vi "dI-dV(V)_two devices_MFLI_MF-MD_K3636B_PK_V4.0_Ja.vi"() -> ()   [LabVIEW 2016]
uses:
  <instrlib>/Keithley 2600 Series/Public/Configure/Source/Configure Source (Limit).vi
  <instrlib>/Keithley 2600 Series/Public/Configure/Source/Configure Source (Range).vi
  <instrlib>/Zurich Instruments LabOne/Public/Configure/ziSetValueDouble.vi
  <instrlib>/Zurich Instruments LabOne/Public/Configure/ziGetValueDemodSampleEx.vi
  <instrlib>/Zurich Instruments LabOne/Zurich Instruments LabOne.lvlib
  <instrlib>/Keithley 2600 Series/Keithley 2600 Series.lvlib
panel:
  in  "MFLI autorange":bool
  in  "MFLI autophase":bool=TRUE
  out "data 2":dbl[](array[numeric])=[5031.359, -0.0019808823515, 7.18983667949342e-11, 8.223089583294991e-06, 8.743473613736861e-06, -0.30000000000000016, -1.500000000000001e-08]
  in  "Tab Control":enum32{"Device 1", "Device 2"}(tab)
  out "dI/dV vs DC Bias (Device 1)":cluster{dbl, "Field Reading":dbl}[](graph)=[{-0.0016781686070000002, "Field Reading"=2.2748202419571386e-06}, {-0.0016578232874999998, "Field Reading"=2.3367028842127987e-06}, {-0.0016344170475, "Field Reading"=2.3324300158885588e-06}, {-0.0016187565549999998, "Field Reading"=2.368210290712901e-06}, {-0.0015966937695, "Field Reading"=2.4050914536005733e-06}, {-0.0015758724415, "Field Reading"=2.462219692201584e-06}, {-0.001552636935, "Field Reading"=2.492132794862598e-06}, {-0.0015335452565, "Field Reading"=2.4689307008136067e-06}, {-0.0015116246024999998, "Field Reading"=2.4182849093288775e-06}, {-0.0014938772125, "Field Reading"=2.3712011536684357e-06}, {-0.001474904835, "Field Reading"=2.336630295077755e-06}, {-0.0014527027135000001, "Field Reading"=2.3489588007080005e-06}, {-0.001433562216, "Field Reading"=2.4000938479599767e-06}, {-0.0014114578835, "Field Reading"=2.476972445250347e-06}, {-0.0013909678065, "Field Reading"=2.4748882698978836e-06}, {-0.0013701705325, "Field Reading"=2.4943669070846246e-06}, {-0.0013500854295, "Field Reading"=2.3374835348545e-06}, {-0.001329588169, "Field Reading"=2.3918021586585987e-06}, {-0.0013049871675, "Field Reading"=2.3538476891368262e-06}, {-0.0012840006455, "Field Reading"=2.3655270828280774e-06}, {-0.0012618388145000002, "Field Reading"=2.3639780156972095e-06}, {-0.00124344113, "Field Reading"=2.403116336754186e-06}, {-0.0012219718954999998, "Field Reading"=2.431417840784851e-06}, {-0.001202953678, "Field Reading"=2.471069543789884e-06}, {-0.0011845934035, "Field Reading"=2.4056313648565487e-06}, {-0.001163120341, "Field Reading"=2.4210561267999395e-06}, {-0.0011410512715000001, "Field Reading"=2.4139294035355594e-06}, {-0.0011204593085, "Field Reading"=2.3566143298824578e-06}, {-0.001099341988, "Field Reading"=2.357179638366921e-06}, {-0.0010774412675, "Field Reading"=2.387342688787914e-06}, {-0.0010571035834999998, "Field Reading"=2.4464943150537807e-06}, {-0.0010358172779999998, "Field Reading"=2.497682003037491e-06}, {-0.0010088930995000001, "Field Reading"=2.4864693695646343e-06}, {-0.0009867399059, "Field Reading"=2.5096665255253005e-06}, {-0.0009655577075500001, "Field Reading"=2.465620761667207e-06}, {-0.0009458661062, "Field Reading"=2.4307695453221525e-06}, {-0.0009252048277999999, "Field Reading"=2.421054638481959e-06}, {-0.00090679080075, "Field Reading"=2.428556545603302e-06}, {-0.0008850208119, "Field Reading"=2.428146478326726e-06}, {-0.0008673084091499999, "Field Reading"=2.49410442618141e-06}, {-0.0008469656851, "Field Reading"=2.490580920504568e-06}, {-0.0008281377888499999, "Field Reading"=2.496431427929007e-06}, {-0.0008051842616000001, "Field Reading"=2.5145014368490632e-06}, {-0.0007834333104, "Field Reading"=2.4783347254970607e-06}, {-0.0007660581869999999, "Field Reading"=2.443329028877877e-06}, {-0.0007436395367500001, "Field Reading"=2.44142699720188e-06}, {-0.0007254273517, "Field Reading"=2.4611120593828642e-06}, {-0.0007057087035499999, "Field Reading"=2.5016309463075904e-06}, {-0.0006887961097, "Field Reading"=2.516924018053863e-06}, {-0.0006729381049, "Field Reading"=2.590030742131985e-06}, {-0.0006516637135499999, "Field Reading"=2.603992917452347e-06}, {-0.00063169264, "Field Reading"=2.604229415404291e-06}, {-0.0006117983212, "Field Reading"=2.606941000307592e-06}, {-0.0006079267094500001, "Field Reading"=2.589576118461254e-06}, {-0.0006042480420000001, "Field Reading"=2.5758610764022937e-06}, {-0.00059714226775, "Field Reading"=2.5869719059328387e-06}, {-0.0005935756073500001, "Field Reading"=2.6167684332302064e-06}, {-0.0005923493795999999, "Field Reading"=2.622151887279586e-06}, {-0.00058669113495, "Field Reading"=2.639268506230056e-06}, {-0.0005840385321, "Field Reading"=2.6325548893594674e-06}, {-0.0005812343410000001, "Field Reading"=2.634813254792392e-06}, {-0.0005774891714999999, "Field Reading"=2.605435851616539e-06}, {-0.00057348596645, "Field Reading"=2.5730920874497637e-06}, {-0.0005712032620500001, "Field Reading"=2.594288346582404e-06}, {-0.0005660910626999998, "Field Reading"=2.6346256844249117e-06}, {-0.0005579502080500001, "Field Reading"=2.6390107964200147e-06}, {-0.0005579058370499999, "Field Reading"=2.6530133586738e-06}, {-0.00055145335495, "Field Reading"=2.647417647039899e-06}, {-0.0005437829652500001, "Field Reading"=2.659094828275176e-06}, {-0.0005425235839, "Field Reading"=2.679548947705164e-06}, {-0.0005357016745499999, "Field Reading"=2.6582071716250706e-06}, {-0.0005345962602500001, "Field Reading"=2.6842337881496388e-06}, {-0.0005288782286999999, "Field Reading"=2.682052233329872e-06}, {-0.0005249209622999999, "Field Reading"=2.674933609281528e-06}, {-0.0005214589899, "Field Reading"=2.714426111664327e-06}, {-0.0005199533409500001, "Field Reading"=2.720132769260274e-06}, {-0.00051627989755, "Field Reading"=2.723672531144842e-06}, {-0.0005109681523000001, "Field Reading"=2.7162779600381256e-06}, {-0.0005068616595000001, "Field Reading"=2.684561849026622e-06}, {-0.00050564747965, "Field Reading"=2.6986704601466846e-06}, {-0.0005019664641, "Field Reading"=2.702091471489977e-06}, {-0.0004979577218, "Field Reading"=2.7119135069852784e-06}, {-0.0004923104790000001, "Field Reading"=2.7570657471800786e-06}, {-0.0004894568168, "Field Reading"=2.7504379280486713e-06}, {-0.00048365580509999995, "Field Reading"=2.7644636045409856e-06}, {-0.0004801527926999999, "Field Reading"=2.7831703035828716e-06}, {-0.00047733695120000003, "Field Reading"=2.7733482137811025e-06}, {-0.00047601134070000004, "Field Reading"=2.7671489265064147e-06}, {-0.00047581607759999994, "Field Reading"=2.783909946368115e-06}, {-0.0004704096427, "Field Reading"=2.801911473608353e-06}, {-0.00046861240325, "Field Reading"=2.8236802071467998e-06}, {-0.00046322419025000003, "Field Reading"=2.8333481922928463e-06}, {-0.0004605137388, "Field Reading"=2.8761025972598264e-06}, {-0.00045492514960000004, "Field Reading"=2.8837078407621434e-06}, {-0.0004529170635, "Field Reading"=2.8934887844165148e-06}, {-0.00045135896890000006, "Field Reading"=2.896673278930621e-06}, {-0.00044494894805, "Field Reading"=2.8860886263753515e-06}, {-0.00044247959965000003, "Field Reading"=2.902846569547315e-06}, {-0.00044029491119999993, "Field Reading"=2.9109838132426387e-06}, {-0.00043641780474999996, "Field Reading"=2.9645674739912844e-06}, {-0.00043149492994999997, "Field Reading"=2.982754927517745e-06}, {-0.0004286056468500001, "Field Reading"=2.990302109847995e-06}, {-0.00042478358424999997, "Field Reading"=3.015337705320556e-06}, {-0.0004225945902000001, "Field Reading"=2.9842607125546776e-06}, {-0.0004184122294, "Field Reading"=2.984506324426212e-06}, {-0.00041357744149999996, "Field Reading"=3.0390464369388424e-06}, {-0.0004111459199000001, "Field Reading"=3.0291665690718033e-06}, {-0.00040689365230000006, "Field Reading"=3.0715937809113967e-06}, {-0.00040518229750000003, "Field Reading"=3.114101950967211e-06}, {-0.0004011455812, "Field Reading"=3.1648742180858055e-06}, {-0.0003964662904500001, "Field Reading"=3.1745671948031264e-06}, {-0.00039702169265, "Field Reading"=3.1774596906502542e-06}, {-0.00039399612740000003, "Field Reading"=3.157372008000181e-06}, {-0.00038918269784999997, "Field Reading"=3.1994110128810866e-06}, {-0.0003864127548, "Field Reading"=3.2376544083055237e-06}, {-0.00038310560055, "Field Reading"=3.281540599918077e-06}, {-0.0003834916401, "Field Reading"=3.3085514260845756e-06}, {-0.0003814061028000001, "Field Reading"=3.30432053588244e-06}, {-0.000375048847, "Field Reading"=3.343056066690764e-06}, {-0.00037155534524999995, "Field Reading"=3.33028660214074e-06}, {-0.00036702173114999995, "Field Reading"=3.3373043766689845e-06}, {-0.0003648478408, "Field Reading"=3.3232910528909814e-06}, {-0.0003592457339, "Field Reading"=3.3456261253236792e-06}, {-0.00035738544415000003, "Field Reading"=3.383381121356372e-06}, {-0.00035428673340000006, "Field Reading"=3.4045550663089754e-06}, {-0.00035342673684999996, "Field Reading"=3.395299738292761e-06}, {-0.00034777238215, "Field Reading"=3.375578582530614e-06}, {-0.0003441009753, "Field Reading"=3.3406980202547656e-06}, {-0.00033877164904999997, "Field Reading"=3.340419604060906e-06}, {-0.00033772544689999995, "Field Reading"=3.2879743278704846e-06}, {-0.00033316558825, "Field Reading"=3.3157345657896806e-06}, {-0.00033273606219999996, "Field Reading"=3.2888005087386516e-06}, {-0.00033209990495, "Field Reading"=3.288887937709162e-06}, {-0.00032745661514999995, "Field Reading"=3.263023003622606e-06}, {-0.0003250379908, "Field Reading"=3.182441976449309e-06}, {-0.00031881736705000003, "Field Reading"=3.127110723048189e-06}, {-0.00031499489720000003, "Field Reading"=3.1017571981904084e-06}, {-0.00031460731355000004, "Field Reading"=2.9992483969271316e-06}, {-0.00030869831080000004, "Field Reading"=2.954708767801396e-06}, {-0.00030794162709999996, "Field Reading"=2.8901718224967945e-06}, {-0.00030571061830000007, "Field Reading"=2.8431408194716333e-06}, {-0.0002990135567, "Field Reading"=2.768940923257753e-06}, {-0.00029867967905, "Field Reading"=2.6817233424575683e-06}, {-0.0002959849753, "Field Reading"=2.5930327791768634e-06}, {-0.00029220280945, "Field Reading"=2.5313375120740387e-06}, {-0.00028515035855000004, "Field Reading"=2.4826260808395303e-06}, {-0.00028006889420000003, "Field Reading"=2.420566117441773e-06}, {-0.0002767854038, "Field Reading"=2.4077559732587833e-06}, {-0.00026997901649999993, "Field Reading"=2.376046906365534e-06}, {-0.0002672423732000001, "Field Reading"=2.3182181599818645e-06}, {-0.00026544306234999997, "Field Reading"=2.2877163561383855e-06}, {-0.00026009267250000004, "Field Reading"=2.2561906511646985e-06}, {-0.00025998314025000007, "Field Reading"=2.220379233291782e-06}, {-0.0002518315652, "Field Reading"=2.2204589017045663e-06}, {-0.0002490530051, "Field Reading"=2.2098376182640844e-06}, {-0.00024523712655, "Field Reading"=2.243689135721626e-06}, {-0.0002388192432, "Field Reading"=2.2614349548247513e-06}, {-0.00023874453295000004, "Field Reading"=2.2605886720515928e-06}, {-0.0002336784888, "Field Reading"=2.28239511710958e-06}, {-0.00022991527609999996, "Field Reading"=2.300911709922007e-06}, {-0.0002271480812, "Field Reading"=2.3194528078580753e-06}, {-0.00022323056190000001, "Field Reading"=2.3197076148652402e-06}, {-0.00021619306005000002, "Field Reading"=2.3290159619604873e-06}, {-0.00021557638660000002, "Field Reading"=2.3484112297882923e-06}, {-0.00020983825865000002, "Field Reading"=2.4240993432233453e-06}, {-0.00020704129859999996, "Field Reading"=2.4591749688146063e-06}, {-0.00020149841305, "Field Reading"=2.4819147229731025e-06}, {-0.00019339191225000002, "Field Reading"=2.496573196748821e-06}, {-0.00019049846375000004, "Field Reading"=2.5458058872022042e-06}, {-0.00018990792505, "Field Reading"=2.575924339023632e-06}, {-0.00018561773995000002, "Field Reading"=2.5816405717962536e-06}, {-0.00018051835035000002, "Field Reading"=2.624016768216242e-06}, {-0.00017305500495, "Field Reading"=2.6974630658947312e-06}, {-0.0001686122808, "Field Reading"=2.7485115767407664e-06}, {-0.00016715574050000002, "Field Reading"=2.765893624967288e-06}, {-0.00016367408255000003, "Field Reading"=2.8022492201742214e-06}, {-0.0001598107689, "Field Reading"=2.8577029550234382e-06}, {-0.00015622802745, "Field Reading"=2.9085152907975607e-06}, {-0.00015515962279999998, "Field Reading"=2.9285918474602912e-06}, {-0.00014715056175, "Field Reading"=3.009552455605472e-06}, {-0.0001454286853, "Field Reading"=3.0350496811641464e-06}, {-0.0001400883418, "Field Reading"=3.031190821614253e-06}, {-0.0001386776494, "Field Reading"=3.0307874089320297e-06}, {-0.00013703432974999997, "Field Reading"=3.0822614418769166e-06}, {-0.00013069768599999998, "Field Reading"=3.1343879307690852e-06}, {-0.00012765424715, "Field Reading"=3.1263704914436776e-06}, {-0.00012263925060000002, "Field Reading"=3.086497529490604e-06}, {-0.00012183433065, "Field Reading"=3.072009972354236e-06}, {-0.00011726607255000002, "Field Reading"=3.086810909815565e-06}, {-0.0001150918153, "Field Reading"=3.0421024014338805e-06}, {-0.00011220979905, "Field Reading"=2.9720511739815787e-06}, {-0.00011021048639999998, "Field Reading"=2.9763858725999805e-06}, {-0.00010715191150000001, "Field Reading"=2.964807577975897e-06}, {-0.0001052300744, "Field Reading"=2.860554609067513e-06}, {-0.00010362509415, "Field Reading"=2.8281332793915137e-06}, {-9.817884581e-05, "Field Reading"=2.7704492440864296e-06}, {-9.5326622965e-05, "Field Reading"=2.6668160951930118e-06}, {-9.468971848000001e-05, "Field Reading"=2.5743842399792543e-06}, {-9.545333745e-05, "Field Reading"=2.5139727238725454e-06}, {-9.706948802000001e-05, "Field Reading"=2.463105093849118e-06}, {-9.473180541000002e-05, "Field Reading"=2.3535738246767888e-06}, {-9.088943867999999e-05, "Field Reading"=2.268291062921381e-06}, {-8.371548238e-05, "Field Reading"=2.066631066064297e-06}, {-8.2325425315e-05, "Field Reading"=2.0216387232900057e-06}, {-8.2863686515e-05, "Field Reading"=1.8705232659793892e-06}, {-8.29676607e-05, "Field Reading"=1.7634877951028684e-06}, {-7.779076009499999e-05, "Field Reading"=1.59138777244819e-06}, {-7.0183610765e-05, "Field Reading"=1.4492529374236303e-06}, {-6.707228585e-05, "Field Reading"=1.2926136683558641e-06}, {-6.248653248499999e-05, "Field Reading"=1.149808285944255e-06}, {-5.5890965495000005e-05, "Field Reading"=9.651270221448368e-07}, {-4.7973332645e-05, "Field Reading"=7.820708706289662e-07}, {-3.921859448e-05, "Field Reading"=6.195401073198032e-07}, {-3.2312716190000004e-05, "Field Reading"=4.6159610908307125e-07}, {-1.8594121749999997e-05, "Field Reading"=3.1684235769834e-07}, {1.6033734839199998e-06, "Field Reading"=1.9384466332408737e-07}, {4.728332178e-05, "Field Reading"=1.2404607316778804e-07}, {0.00016402269849999997, "Field Reading"=1.1311076597304693e-07}, {0.00023340214154999998, "Field Reading"=1.35852454274743e-07}, {0.00025888455309999996, "Field Reading"=2.3237881305734114e-07}, {0.00027773405205, "Field Reading"=3.54983025250113e-07}, {0.00029051388449999994, "Field Reading"=5.041978002207515e-07}, {0.0002976315571, "Field Reading"=6.619464306603345e-07}, {0.00030398340470000004, "Field Reading"=8.146307576296449e-07}, {0.00030901783514999996, "Field Reading"=9.082071479107701e-07}, {0.00031756279870000004, "Field Reading"=1.1090702382910265e-06}, {0.0003220707941, "Field Reading"=1.1950649011174367e-06}, {0.00032795834225000003, "Field Reading"=1.2069447013135315e-06}, {0.0003331217398999999, "Field Reading"=1.3297858715175994e-06}, {0.00033592983009999997, "Field Reading"=1.4014874837727866e-06}, {0.00033849589635, "Field Reading"=1.4369617582755556e-06}, {0.0003458102554, "Field Reading"=1.506035011640962e-06}, {0.0003481475298, "Field Reading"=1.5687227562455348e-06}, {0.0003480479931, "Field Reading"=1.5766096984561574e-06}, {0.0003534967314, "Field Reading"=1.5999829001629195e-06}, {0.0003572715896500001, "Field Reading"=1.6643167201025153e-06}, {0.00035776291469999996, "Field Reading"=1.6652335253252737e-06}, {0.0003607961883, "Field Reading"=1.6612564436585664e-06}, {0.0003636120904, "Field Reading"=1.675888679569357e-06}, {0.00036818265540000005, "Field Reading"=1.6730081523184478e-06}, {0.00037362200355, "Field Reading"=1.670846518835472e-06}, {0.0003735467712, "Field Reading"=1.6759437814247057e-06}, {0.00037906393304999996, "Field Reading"=1.6546069206293473e-06}, {0.0003784099651, "Field Reading"=1.626087574488874e-06}, {0.0003820362876, "Field Reading"=1.6278703398385884e-06}, {0.00038452126115, "Field Reading"=1.603612062221844e-06}, {0.0003885724355, "Field Reading"=1.5943163978338533e-06}, {0.00039126967175, "Field Reading"=1.5867210449901996e-06}, {0.0003975379796000001, "Field Reading"=1.5555441704337225e-06}, {0.00040107856935, "Field Reading"=1.536530641959993e-06}, {0.0004052368369999999, "Field Reading"=1.5063117864593086e-06}, {0.0004046776544, "Field Reading"=1.511884299590203e-06}, {0.00041075511219999995, "Field Reading"=1.4831125730190307e-06}, {0.0004151184367, "Field Reading"=1.472534501292197e-06}, {0.00041891397965000004, "Field Reading"=1.4613192371032018e-06}, {0.00041985447225, "Field Reading"=1.4349583649137389e-06}, {0.0004204693849500001, "Field Reading"=1.4062032318763324e-06}, {0.00042510339585000005, "Field Reading"=1.4202530516020666e-06}, {0.00042854531935000007, "Field Reading"=1.3944115795476666e-06}, {0.00043297750585, "Field Reading"=1.377396202393783e-06}, {0.0004352429830999999, "Field Reading"=1.3683939893944844e-06}, {0.00043975237154999993, "Field Reading"=1.3726338470753034e-06}, {0.000446042927, "Field Reading"=1.3619563481756559e-06}, {0.0004486403547499999, "Field Reading"=1.3348845495134537e-06}, {0.00045554409329999994, "Field Reading"=1.3500331019691104e-06}, {0.0004604035046499999, "Field Reading"=1.3431656272677353e-06}, {0.00046818487054999994, "Field Reading"=1.3585531402549034e-06}, {0.00047523929064999997, "Field Reading"=1.3346477762105235e-06}, {0.00048154575775000006, "Field Reading"=1.3659751609650056e-06}, {0.0004884181508499998, "Field Reading"=1.45712088171546e-06}, {0.0004938996670000001, "Field Reading"=1.5317145721155254e-06}, {0.0005003480080999999, "Field Reading"=1.6303249953289446e-06}, {0.0005075438409, "Field Reading"=1.770024508985041e-06}, {0.0005141938976499999, "Field Reading"=1.8669046977430722e-06}, {0.0005188101553499999, "Field Reading"=2.0169232159425276e-06}, {0.0005248727863500001, "Field Reading"=2.1282289832338904e-06}, {0.0005274987118, "Field Reading"=2.2699458394928817e-06}, {0.0005344199591, "Field Reading"=2.463912264839736e-06}, {0.0005386740678, "Field Reading"=2.6124791135069678e-06}, {0.0005427686072, "Field Reading"=2.759526866639913e-06}, {0.0005444155226499999, "Field Reading"=2.9448155424906587e-06}, {0.0005435634498499999, "Field Reading"=3.0716319517988875e-06}, {0.0005485915596999999, "Field Reading"=3.2424644642738137e-06}, {0.0005501732642, "Field Reading"=3.3446895985090555e-06}, {0.00055458526355, "Field Reading"=3.3532927472371605e-06}, {0.0005549940035999999, "Field Reading"=3.4852144896479896e-06}, {0.00056104059655, "Field Reading"=3.577588288160979e-06}, {0.0005650095690000001, "Field Reading"=3.6325875579915108e-06}, {0.00056324549495, "Field Reading"=3.7119141670088987e-06}, {0.00056634243855, "Field Reading"=3.768452015870618e-06}, {0.0005671589003999999, "Field Reading"=3.758016491766289e-06}, {0.0005706185166500001, "Field Reading"=3.8161718129661095e-06}, {0.0005698794003499999, "Field Reading"=3.843699806662378e-06}, {0.00057325087445, "Field Reading"=3.923597190003678e-06}, {0.0005751604092500001, "Field Reading"=3.983873406127606e-06}, {0.0005762745515000001, "Field Reading"=3.927155055777594e-06}, {0.0005806333359, "Field Reading"=3.947559855594881e-06}, {0.0005851516545000001, "Field Reading"=3.997729497137463e-06}, {0.0005854238656500001, "Field Reading"=3.935526839117798e-06}, {0.00058721746155, "Field Reading"=3.926583508893878e-06}, {0.0005901182206499999, "Field Reading"=3.93064936152259e-06}, {0.0005957065574000001, "Field Reading"=3.907110931655071e-06}, {0.00059421468415, "Field Reading"=3.862135582908162e-06}, {0.0005934460853999999, "Field Reading"=3.821217161735101e-06}, {0.00060261118585, "Field Reading"=3.7982152303450205e-06}, {0.0006051394554500001, "Field Reading"=3.793064976418888e-06}, {0.0006079941955500001, "Field Reading"=3.746324285259505e-06}, {0.0006081191610999998, "Field Reading"=3.6857500611095683e-06}, {0.00061038616585, "Field Reading"=3.678100479527705e-06}, {0.0006100890781999999, "Field Reading"=3.675811428422848e-06}, {0.00061155401225, "Field Reading"=3.6368507993996494e-06}, {0.0006154215189000001, "Field Reading"=3.6134872163081277e-06}, {0.00061825350855, "Field Reading"=3.5087198549170332e-06}, {0.0006252284634500001, "Field Reading"=3.503800654052068e-06}, {0.00063172252175, "Field Reading"=3.4530405807113654e-06}, {0.0006330941998, "Field Reading"=3.426565880337807e-06}, {0.0006344631709000001, "Field Reading"=3.431877186913347e-06}, {0.00063394018725, "Field Reading"=3.420896791724277e-06}, {0.00063832676185, "Field Reading"=3.3788663889520888e-06}, {0.0006394003013999999, "Field Reading"=3.321477155515018e-06}, {0.0006414651024000001, "Field Reading"=3.279957660331102e-06}, {0.00064639568185, "Field Reading"=3.2723708907740863e-06}, {0.0006434985454, "Field Reading"=3.2474871178487876e-06}, {0.00064798426365, "Field Reading"=3.2232339793081447e-06}, {0.0006476101279, "Field Reading"=3.2046998052240347e-06}, {0.0006538107537499999, "Field Reading"=3.2096807354486713e-06}, {0.0006571143322, "Field Reading"=3.1923339839698905e-06}, {0.0006618326586, "Field Reading"=3.1608665895277192e-06}, {0.0006640560491499999, "Field Reading"=3.125145566994127e-06}, {0.0006640121938, "Field Reading"=3.106728834435098e-06}, {0.00066895752485, "Field Reading"=3.078858162495081e-06}, {0.0006735744178499999, "Field Reading"=3.0898692437445493e-06}, {0.0006786077272, "Field Reading"=3.0667631336552088e-06}, {0.0006823110916, "Field Reading"=3.0612618151696445e-06}, {0.00068539706775, "Field Reading"=3.0521771487713005e-06}, {0.0006909548427, "Field Reading"=3.0318929796186587e-06}, {0.00069209169655, "Field Reading"=2.960316750779192e-06}, {0.0006913875720499999, "Field Reading"=2.9620217068520062e-06}, {0.0006929332142, "Field Reading"=2.934049062457863e-06}, {0.0007015408406999999, "Field Reading"=2.9373905943054486e-06}, {0.0007048490830999999, "Field Reading"=2.9258962244966193e-06}, {0.00070863480745, "Field Reading"=2.94516701087845e-06}, {0.0007094327866, "Field Reading"=2.906763489794304e-06}, {0.0007144370181999999, "Field Reading"=2.8982141228867684e-06}, {0.0007169354648, "Field Reading"=2.887065788136323e-06}, {0.0007165005145000001, "Field Reading"=2.8687855823386107e-06}, {0.0007191513395, "Field Reading"=2.8217837143788857e-06}, {0.0007219917239999999, "Field Reading"=2.8148218578639517e-06}, {0.0007247388581999999, "Field Reading"=2.8391630821091868e-06}, {0.0007289080057999999, "Field Reading"=2.8287795831822896e-06}, {0.0007477472021500001, "Field Reading"=2.7904825063564608e-06}, {0.0007663384343500001, "Field Reading"=2.7762143102645227e-06}, {0.0007823339620000001, "Field Reading"=2.7312320807778656e-06}, {0.0008013025004500001, "Field Reading"=2.7061417313295764e-06}, {0.0008185362253500001, "Field Reading"=2.649309826181418e-06}, {0.0008333156628, "Field Reading"=2.5989488008987505e-06}, {0.0008536235817999999, "Field Reading"=2.5842270578763263e-06}, {0.0008729350676499999, "Field Reading"=2.5675826801701575e-06}, {0.00089402353875, "Field Reading"=2.583983849242866e-06}, {0.000912802295, "Field Reading"=2.576167715205063e-06}, {0.0009340839024999999, "Field Reading"=2.58408927877769e-06}, {0.000950597861, "Field Reading"=2.5720501383586775e-06}, {0.0009710496542499999, "Field Reading"=2.5211974645186055e-06}, {0.0009906135872999999, "Field Reading"=2.4975164492764623e-06}, {0.0010087428499999998, "Field Reading"=2.4623250283252237e-06}, {0.0010279227815000003, "Field Reading"=2.4717321825411283e-06}, {0.0010482391604999999, "Field Reading"=2.4780712839942525e-06}, {0.001068571693, "Field Reading"=2.5116904644736813e-06}, {0.0010859524090000002, "Field Reading"=2.5341028664772476e-06}, {0.0011067198759999997, "Field Reading"=2.484916773194556e-06}, {0.0011301505405000001, "Field Reading"=2.4790183725578907e-06}, {0.0011512843585000001, "Field Reading"=2.442859179327604e-06}, {0.0011680863685, "Field Reading"=2.403572334977321e-06}, {0.0011878621009999998, "Field Reading"=2.3743233554801796e-06}, {0.0012100071925, "Field Reading"=2.4005668706919355e-06}, {0.0012330234169999998, "Field Reading"=2.4300677607007184e-06}, {0.0012559936485, "Field Reading"=2.4583820297258462e-06}, {0.0012739046659999997, "Field Reading"=2.4657461078298674e-06}, {0.0012962089709999999, "Field Reading"=2.464799019945674e-06}, {0.0013147082255, "Field Reading"=2.4397960642520266e-06}, {0.0013346944755, "Field Reading"=2.3907180849033875e-06}, {0.0013575627510000001, "Field Reading"=2.3556311205015775e-06}, {0.0013759980585, "Field Reading"=2.3621624456203644e-06}, {0.0014015571235, "Field Reading"=2.4003257186183773e-06}, {0.0014176177080000001, "Field Reading"=2.4519116905246865e-06}, {0.0014334223479999999, "Field Reading"=2.4830274034937014e-06}, {0.001453914637, "Field Reading"=2.495946496225912e-06}, {0.0014786366844999998, "Field Reading"=2.4620252349713466e-06}]
  out "DC Voltage (V)":dbl=0.0014786366844999998
  out "dI (A)":dbl=2.35323775186076e-11
  out "dV (V)":dbl=9.558138228782806e-06
  out "dI/dV (ohm)":dbl=2.4620252349713466e-06
  out "Vset (V)":dbl=-0.30000000000000016
  in  "Nanovoltmeter 2182A VISA (Device1)":refnum<visa-resource-name>="GPIB0::7::INSTR"
  in  "MFLI Device 1 Address\n(connected to Channel A of K2635B)":string="DEV4382"
  in  "File Name Device 1":string="013_MA2158_STS_[Dev90]_baseT_2T(89.25deg)_measureX_35uV_7.919Hz_ground_100xaverage_finescan"
  in  "From 1":dbl[](array[numeric])=[0.41, 0.15, 0.013, -0.024, -0.11] min=-3000.0 max=3000.0 format="%.2e"
  in  "To 1":dbl[](array[numeric])=[0.15, 0.013, -0.024, -0.11, -0.304] min=-3000.0 max=3000.0 format="%.2e"
  in  "Step 1":dbl[](array[numeric])=[0.005, 0.001, 0.0005, 0.001, 0.005] min=-3000.0 max=3000.0 format="%.1e"
  in  "Resistance used for DC (Device 1) (ohm)":dbl=100000000.0 format="%#_13g"
  in  "DC Voltage averaging (Device 1)":dbl=20.0 format="%#_13g"
  in  "MFLI Averaging (Device1)":dbl=100.0 format="%#_13g"
  in  "MFLI Device 1 Delay (s)":dbl=4.0
  in  "MFLI Device 2 Address\n(connected to Channel B of K2635B)":string="DEV4496"
  in  "Resistance used for DC (ohm) 2":dbl=20000000.0 format="%#_13g"
  in  "Nanovoltmeter 2182a VISA (Device 2)":refnum<visa-resource-name>="GPIB0::4::INSTR"
  in  "File Name Device 2":string="014_MA2158_STS_[Dev150]_baseT_2T(89.25deg)_measureX_35uV_17.7777Hz_ground_100xaverage_finescan"
  in  "MFLI Device 2 Delay (s)":dbl=4.0
  in  "From 3":dbl[](array[numeric])=[0.304, 0.12, 0.013, -0.024, -0.11] min=-3000.0 max=3000.0 format="%.2e"
  in  "To 3":dbl[](array[numeric])=[0.12, 0.013, -0.024, -0.11, -0.304] min=-3000.0 max=3000.0 format="%.2e"
  in  "Step 3":dbl[](array[numeric])=[0.005, 0.001, 0.0005, 0.001, 0.005] min=-3000.0 max=3000.0 format="%.1e"
  out "dI/dV vs DC Bias (Device 2)":cluster{dbl, "Field Reading":dbl}[](graph)=[{0.0016771856900000004, "Field Reading"=8.462398793511336e-06}, {0.0016502059324999998, "Field Reading"=8.617850250648297e-06}, {0.001621715692, "Field Reading"=8.826717050364379e-06}, {0.001590235113, "Field Reading"=8.87925703203224e-06}, {0.0015640726564999999, "Field Reading"=8.710217701828672e-06}, {0.0015307174545, "Field Reading"=8.756431672896166e-06}, {0.0015029417390000001, "Field Reading"=8.950063980264438e-06}, {0.0014736772204999998, "Field Reading"=8.819132606847237e-06}, {0.0014452695330000001, "Field Reading"=8.654747934089483e-06}, {0.0014217917355, "Field Reading"=8.74717871411561e-06}, {0.0013917154325, "Field Reading"=8.925404962491958e-06}, {0.0013659046310000001, "Field Reading"=8.787036293957644e-06}, {0.0013345645625, "Field Reading"=8.698969305361074e-06}, {0.0013059019409999999, "Field Reading"=8.924580683037864e-06}, {0.0012791606195, "Field Reading"=8.808035222811866e-06}, {0.0012484019105000002, "Field Reading"=8.73949960008534e-06}, {0.0012206773195, "Field Reading"=8.81417587393598e-06}, {0.0011897090395000002, "Field Reading"=8.92919081795301e-06}, {0.0011594695149999999, "Field Reading"=8.77715595107947e-06}, {0.0011349323645, "Field Reading"=8.757665692069127e-06}, {0.0011052842289999997, "Field Reading"=8.841569911422271e-06}, {0.0010771110189999999, "Field Reading"=8.87949145553544e-06}, {0.001049195784, "Field Reading"=8.80317868790248e-06}, {0.0010202332690000002, "Field Reading"=8.853718917375634e-06}, {0.0009915124328, "Field Reading"=9.05548462195946e-06}, {0.0009645905549, "Field Reading"=8.852712737771398e-06}, {0.0009364647443500001, "Field Reading"=8.876383906463695e-06}, {0.0009088378339, "Field Reading"=8.898791841999551e-06}, {0.0008810276324000001, "Field Reading"=8.981176599163999e-06}, {0.00085048161755, "Field Reading"=8.919275931848804e-06}, {0.00082544772825, "Field Reading"=8.930525980231723e-06}, {0.0007980101465999999, "Field Reading"=9.054290167151437e-06}, {0.000768123579, "Field Reading"=8.943876374597851e-06}, {0.0007411195732, "Field Reading"=9.03837270068478e-06}, {0.00071619687135, "Field Reading"=9.14159207700073e-06}, {0.0006895219277000001, "Field Reading"=9.19157841114815e-06}, {0.0006656113926, "Field Reading"=9.167940152955321e-06}, {0.0006448383220000001, "Field Reading"=9.267631760838387e-06}, {0.00063894485435, "Field Reading"=9.306555702003775e-06}, {0.0006353674875, "Field Reading"=9.294900449834778e-06}, {0.0006276397279000001, "Field Reading"=9.249246789232744e-06}, {0.00062374287175, "Field Reading"=9.294123852878546e-06}, {0.0006187933342500002, "Field Reading"=9.397633057837105e-06}, {0.00060947688215, "Field Reading"=9.32537231318e-06}, {0.00060446504685, "Field Reading"=9.35978662690125e-06}, {0.00060003803105, "Field Reading"=9.45650527378569e-06}, {0.0005948330642999999, "Field Reading"=9.44565985342106e-06}, {0.0005890849741999999, "Field Reading"=9.353604778759287e-06}, {0.0005786774389499999, "Field Reading"=9.405786150624375e-06}, {0.0005753718466999999, "Field Reading"=9.543448065752312e-06}, {0.0005697526635, "Field Reading"=9.467405631356763e-06}, {0.00056509829875, "Field Reading"=9.454967664414277e-06}, {0.0005581239462999999, "Field Reading"=9.557544186655155e-06}, {0.0005526130854999999, "Field Reading"=9.562871414096004e-06}, {0.0005429059492000001, "Field Reading"=9.55863401155072e-06}, {0.00053623342815, "Field Reading"=9.601911015531037e-06}, {0.0005300931349499999, "Field Reading"=9.58993635065981e-06}, {0.0005278333883500001, "Field Reading"=9.621439680855302e-06}, {0.00052323914405, "Field Reading"=9.618090337769185e-06}, {0.0005185157989, "Field Reading"=9.710346414401627e-06}, {0.00051280316605, "Field Reading"=9.78893398781927e-06}, {0.00050671528865, "Field Reading"=9.76895330936452e-06}, {0.0005029942170999999, "Field Reading"=9.745234800525845e-06}, {0.00049592673775, "Field Reading"=9.82228996289577e-06}, {0.0004934526097, "Field Reading"=9.855750637386827e-06}, {0.00048304480394999996, "Field Reading"=9.88665733592811e-06}, {0.000474863974, "Field Reading"=9.958193277991383e-06}, {0.00046902268959999997, "Field Reading"=9.965312645114401e-06}, {0.00046696993295000004, "Field Reading"=9.96616954127336e-06}, {0.00046532135094999995, "Field Reading"=1.001910639089078e-05}, {0.00045974837069999994, "Field Reading"=1.0092781598783261e-05}, {0.0004552897543, "Field Reading"=1.011576892508962e-05}, {0.00045133895555, "Field Reading"=1.0126382465110586e-05}, {0.00045014077925000005, "Field Reading"=1.0194694643913358e-05}, {0.00044539740690000007, "Field Reading"=1.0326474360273323e-05}, {0.00044109899724999993, "Field Reading"=1.0380371547812062e-05}, {0.0004385090055, "Field Reading"=1.0369642979391752e-05}, {0.00043379648275, "Field Reading"=1.044321413856346e-05}, {0.0004289066501500001, "Field Reading"=1.0485550994514976e-05}, {0.0004210223042, "Field Reading"=1.0577777738567291e-05}, {0.00041600563535, "Field Reading"=1.0637331087043215e-05}, {0.00041495100785000005, "Field Reading"=1.0715874392231338e-05}, {0.00041034747955, "Field Reading"=1.0763302646881858e-05}, {0.0004101617789499999, "Field Reading"=1.0796004912129737e-05}, {0.00040352732930000007, "Field Reading"=1.09244875199915e-05}, {0.00039698713025, "Field Reading"=1.1051565537418268e-05}, {0.00039361926089999996, "Field Reading"=1.1079522004774359e-05}, {0.00038994246729999997, "Field Reading"=1.1180616352896856e-05}, {0.00038321697945, "Field Reading"=1.1254141428780924e-05}, {0.0003805111036, "Field Reading"=1.1337952432620073e-05}, {0.0003760655413, "Field Reading"=1.1385949354066463e-05}, {0.00037298759629999996, "Field Reading"=1.156363765275925e-05}, {0.00036903100809999997, "Field Reading"=1.160731206274308e-05}, {0.00036339895105, "Field Reading"=1.1707855191516176e-05}, {0.0003552188896, "Field Reading"=1.1763510908881959e-05}, {0.00035454741410000004, "Field Reading"=1.1933682445473304e-05}, {0.0003493671564500001, "Field Reading"=1.19119548587962e-05}, {0.0003452999583000001, "Field Reading"=1.2010167340324472e-05}, {0.0003425712415, "Field Reading"=1.2032822363039686e-05}, {0.00033958025874999997, "Field Reading"=1.2008299537711947e-05}, {0.00033495246764999996, "Field Reading"=1.2017953259822465e-05}, {0.00033076530565, "Field Reading"=1.2036006619958021e-05}, {0.00032794951075000003, "Field Reading"=1.1929906698085958e-05}, {0.0003202158053, "Field Reading"=1.1966466882279645e-05}, {0.00031827374385000004, "Field Reading"=1.1871958729314474e-05}, {0.0003149108825, "Field Reading"=1.1731991365250255e-05}, {0.00031234787985, "Field Reading"=1.1600667200839073e-05}, {0.00031179938715, "Field Reading"=1.1422721931068642e-05}, {0.00030325476725, "Field Reading"=1.1245563339570872e-05}, {0.00030198047710000006, "Field Reading"=1.0998918839142212e-05}, {0.00029634825874999993, "Field Reading"=1.0785492542100792e-05}, {0.0002924240922, "Field Reading"=1.052462421296895e-05}, {0.00028445265299999997, "Field Reading"=1.0243049649746367e-05}, {0.00028260852125000003, "Field Reading"=1.0040609815888272e-05}, {0.0002783540092, "Field Reading"=9.757823508440813e-06}, {0.00027196160444999996, "Field Reading"=9.473957700176925e-06}, {0.00026709579575000004, "Field Reading"=9.25717499307455e-06}, {0.0002580205054, "Field Reading"=9.039270083404435e-06}, {0.00025446780885, "Field Reading"=8.780332657921238e-06}, {0.0002469900989, "Field Reading"=8.610926569002035e-06}, {0.00023916655970000002, "Field Reading"=8.509371305413043e-06}, {0.00022920085745, "Field Reading"=8.428566838329146e-06}, {0.0002245226408, "Field Reading"=8.351069193473486e-06}, {0.00021618390469999995, "Field Reading"=8.277735456821629e-06}, {0.00021130762979999998, "Field Reading"=8.36995744738291e-06}, {0.00020150083074999998, "Field Reading"=8.364039853257106e-06}, {0.0001983421883, "Field Reading"=8.394150124065383e-06}, {0.00019280479490000002, "Field Reading"=8.492360778364317e-06}, {0.0001830640891, "Field Reading"=8.620923286542283e-06}, {0.00018242040090000002, "Field Reading"=8.698806203386917e-06}, {0.00017728712935, "Field Reading"=8.843266311316334e-06}, {0.00017195948465, "Field Reading"=8.956124728066143e-06}, {0.0001677756752, "Field Reading"=9.164571041429809e-06}, {0.0001625379775, "Field Reading"=9.295868168359383e-06}, {0.00015508999125000002, "Field Reading"=9.425499652064013e-06}, {0.00015060362275, "Field Reading"=9.59294606347476e-06}, {0.00014632609639999997, "Field Reading"=9.823607682343675e-06}, {0.00013901595925, "Field Reading"=9.998318412077204e-06}, {0.00013444025575, "Field Reading"=1.0182895013077408e-05}, {0.0001296452741, "Field Reading"=1.031522173616421e-05}, {0.00012500901195, "Field Reading"=1.0500508372538445e-05}, {0.00012104320899999999, "Field Reading"=1.0550840196122307e-05}, {0.00011156888045000002, "Field Reading"=1.0672966455461552e-05}, {0.00011000201460000002, "Field Reading"=1.0725845820955066e-05}, {0.00010234320485000002, "Field Reading"=1.064071656566374e-05}, {0.0001029836192, "Field Reading"=1.0649664170941785e-05}, {9.758650826499999e-05, "Field Reading"=1.0533822612272307e-05}, {9.777142439499999e-05, "Field Reading"=1.0558615481619498e-05}, {9.6236653105e-05, "Field Reading"=1.0507870217947494e-05}, {9.203636646500001e-05, "Field Reading"=1.0366771989682448e-05}, {8.896572963e-05, "Field Reading"=1.0241387157632407e-05}, {8.4588023745e-05, "Field Reading"=1.018341496154298e-05}, {8.713646094999999e-05, "Field Reading"=9.964793328528473e-06}, {8.630083548e-05, "Field Reading"=9.830494982006011e-06}, {8.1552566485e-05, "Field Reading"=9.636378199029291e-06}, {8.108748244000001e-05, "Field Reading"=9.431625706333647e-06}, {7.861053252e-05, "Field Reading"=9.170053414579016e-06}, {7.677426311500001e-05, "Field Reading"=8.88499248372687e-06}, {7.244821059000001e-05, "Field Reading"=8.546509053630047e-06}, {7.078400487999999e-05, "Field Reading"=8.182628599637404e-06}, {6.303654371e-05, "Field Reading"=7.869199984478325e-06}, {6.3401604995e-05, "Field Reading"=7.33126832217029e-06}, {6.020828628999999e-05, "Field Reading"=6.811477686200212e-06}, {5.174279605999999e-05, "Field Reading"=6.182430678449056e-06}, {5.0106775155e-05, "Field Reading"=5.601063744100781e-06}, {4.663204943e-05, "Field Reading"=4.890542285105519e-06}, {3.8209257260000005e-05, "Field Reading"=4.206825611258721e-06}, {3.2900075805e-05, "Field Reading"=3.4123685760339093e-06}, {2.3037074555e-05, "Field Reading"=2.79866295668679e-06}, {9.1368322125e-06, "Field Reading"=2.0329323659389314e-06}, {-5.74332000045e-06, "Field Reading"=1.3519121629424724e-06}, {-3.3539505455e-05, "Field Reading"=7.421247557554652e-07}, {-7.1793480065e-05, "Field Reading"=2.669162113533685e-07}, {-0.00020208870320000003, "Field Reading"=1.7983425829912847e-07}, {-0.00025300462465000005, "Field Reading"=5.41248467035181e-07}, {-0.00028050621439999995, "Field Reading"=1.0612257650538083e-06}, {-0.00029734474035, "Field Reading"=1.6412289293857427e-06}, {-0.0003125041635, "Field Reading"=2.2266634826373623e-06}, {-0.00032340798075000004, "Field Reading"=2.7965965752678606e-06}, {-0.0003379056426, "Field Reading"=3.2847943381482522e-06}, {-0.00034679944300000003, "Field Reading"=3.763707292597035e-06}, {-0.00035459496485, "Field Reading"=4.203686082852709e-06}, {-0.00035472971725000003, "Field Reading"=4.522119935408054e-06}, {-0.00036532942815, "Field Reading"=4.882774993730991e-06}, {-0.0003701372254, "Field Reading"=5.151186474145035e-06}, {-0.00037205704815, "Field Reading"=5.330610472298436e-06}, {-0.00037677052200000004, "Field Reading"=5.4914101970531455e-06}, {-0.00038004859354999997, "Field Reading"=5.5855896598693915e-06}, {-0.0003848553823, "Field Reading"=5.668731204818231e-06}, {-0.00038802120680000003, "Field Reading"=5.719309782402168e-06}, {-0.0003940912248, "Field Reading"=5.695560956964821e-06}, {-0.00040040439619999993, "Field Reading"=5.723483367352867e-06}, {-0.00040440363165, "Field Reading"=5.698272810361427e-06}, {-0.00040880195265, "Field Reading"=5.67596100427043e-06}, {-0.00040893651595, "Field Reading"=5.593543824039489e-06}, {-0.00041848630304999995, "Field Reading"=5.530745125706387e-06}, {-0.00041961408319999996, "Field Reading"=5.504624047636624e-06}, {-0.00042378206089999993, "Field Reading"=5.4114894785326846e-06}, {-0.00042891714139999996, "Field Reading"=5.3455170828858e-06}, {-0.00042574521970000005, "Field Reading"=5.255952005991952e-06}, {-0.0004325055203, "Field Reading"=5.220381156997152e-06}, {-0.00043767619475, "Field Reading"=5.161949098751467e-06}, {-0.0004411910198, "Field Reading"=5.096296975916308e-06}, {-0.00044556040965, "Field Reading"=5.037484174951122e-06}, {-0.00045731114510000006, "Field Reading"=5.007480995831883e-06}, {-0.00045934146039999996, "Field Reading"=4.953051680029272e-06}, {-0.00047054122600000007, "Field Reading"=4.959765418521088e-06}, {-0.00047279099020000007, "Field Reading"=4.973699015141517e-06}, {-0.00047823019885000006, "Field Reading"=4.997418608552457e-06}, {-0.00048476093325, "Field Reading"=4.994483054105246e-06}, {-0.00048582291915000005, "Field Reading"=5.074757952663873e-06}, {-0.0004885880974, "Field Reading"=5.121932290810572e-06}, {-0.0004930843359500001, "Field Reading"=5.24361492827317e-06}, {-0.00049563354595, "Field Reading"=5.368609901778681e-06}, {-0.0004993021547999999, "Field Reading"=5.465915017089052e-06}, {-0.0005045761451999999, "Field Reading"=5.672313724610649e-06}, {-0.00051127457365, "Field Reading"=5.833892293469606e-06}, {-0.00051552538715, "Field Reading"=6.05442518229462e-06}, {-0.00051716665835, "Field Reading"=6.297408978676904e-06}, {-0.0005238966327, "Field Reading"=6.802698251294797e-06}, {-0.0005334525741, "Field Reading"=7.392110784393784e-06}, {-0.0005406813666999999, "Field Reading"=8.06118095243527e-06}, {-0.0005465057531, "Field Reading"=8.691377048837602e-06}, {-0.00055290445735, "Field Reading"=9.351205003661786e-06}, {-0.0005560649302999999, "Field Reading"=9.865573990476005e-06}, {-0.0005640491874499999, "Field Reading"=1.0608119814319428e-05}, {-0.0005666129156, "Field Reading"=1.1032226052059645e-05}, {-0.0005688291365999999, "Field Reading"=1.1555591910128647e-05}, {-0.00056902355955, "Field Reading"=1.2051157839430144e-05}, {-0.0005769350082, "Field Reading"=1.2437387417086596e-05}, {-0.0005856075502999999, "Field Reading"=1.2704577115817795e-05}, {-0.000586783283, "Field Reading"=1.2996814886897142e-05}, {-0.00058692203855, "Field Reading"=1.3238806062871321e-05}, {-0.0005941557748999999, "Field Reading"=1.3440439579396907e-05}, {-0.0005983973591, "Field Reading"=1.3587223657398136e-05}, {-0.00060206952005, "Field Reading"=1.3673079779226505e-05}, {-0.0006045420065499999, "Field Reading"=1.3838119021058409e-05}, {-0.0006124162244000001, "Field Reading"=1.3828633848680698e-05}, {-0.0006151569393500001, "Field Reading"=1.3838639931063396e-05}, {-0.0006174305633500001, "Field Reading"=1.3779989806594412e-05}, {-0.00062205551475, "Field Reading"=1.3808683449022883e-05}, {-0.00062665060015, "Field Reading"=1.3760088067492035e-05}, {-0.00062775150285, "Field Reading"=1.370345513486496e-05}, {-0.00063439890175, "Field Reading"=1.3496704473598479e-05}, {-0.0006453107542, "Field Reading"=1.3509995340482848e-05}, {-0.0006454007169, "Field Reading"=1.332851624348292e-05}, {-0.0006504702849500001, "Field Reading"=1.3235615320021187e-05}, {-0.00065683893615, "Field Reading"=1.3022045177512368e-05}, {-0.0006578808655, "Field Reading"=1.3016189146409095e-05}, {-0.0006652263428, "Field Reading"=1.284081975728515e-05}, {-0.0006636386794999999, "Field Reading"=1.263450929871561e-05}, {-0.00066599836165, "Field Reading"=1.254847892135884e-05}, {-0.0006707491693, "Field Reading"=1.2424565832171125e-05}, {-0.0006759197118500001, "Field Reading"=1.2289635763362937e-05}, {-0.0006777452528, "Field Reading"=1.2083486062836349e-05}, {-0.0006816006327, "Field Reading"=1.2042692230147519e-05}, {-0.00068830592625, "Field Reading"=1.1933756606888504e-05}, {-0.00069296477275, "Field Reading"=1.1815279717152957e-05}, {-0.0007010242080000001, "Field Reading"=1.1670516089663457e-05}, {-0.0007098843572499999, "Field Reading"=1.1591811399614844e-05}, {-0.0007147816445499998, "Field Reading"=1.1432527768956521e-05}, {-0.0007202839017499999, "Field Reading"=1.1376671511027448e-05}, {-0.00072260259615, "Field Reading"=1.1243519204887838e-05}, {-0.00072318690035, "Field Reading"=1.1240313926361627e-05}, {-0.0007266260707000001, "Field Reading"=1.1144388565382625e-05}, {-0.0007321243502999998, "Field Reading"=1.1018357826764924e-05}, {-0.00073345156815, "Field Reading"=1.0941929670074046e-05}, {-0.0007342750678500001, "Field Reading"=1.0839587860782853e-05}, {-0.00074190651615, "Field Reading"=1.0740233588320697e-05}, {-0.000747063905, "Field Reading"=1.0715674962811745e-05}, {-0.0007526868720000001, "Field Reading"=1.0675573004793438e-05}, {-0.0007559988450500002, "Field Reading"=1.0644695615647722e-05}, {-0.0007628911484499998, "Field Reading"=1.0489325523449371e-05}, {-0.0007695125547, "Field Reading"=1.0488300117744357e-05}, {-0.00077210940395, "Field Reading"=1.0464457965717215e-05}, {-0.0007766496880499999, "Field Reading"=1.0362519805104074e-05}, {-0.0007807587708000001, "Field Reading"=1.031612920470413e-05}, {-0.0007870510644499999, "Field Reading"=1.0269912494698967e-05}, {-0.0007947768073000001, "Field Reading"=1.0185386535538703e-05}, {-0.0007981852819000001, "Field Reading"=1.0179700949512421e-05}, {-0.0008000154728, "Field Reading"=1.0164200259498789e-05}, {-0.0008042754119, "Field Reading"=1.0107521181120057e-05}, {-0.0008067674517999999, "Field Reading"=1.0034567355523803e-05}, {-0.00081466860945, "Field Reading"=9.999696239398774e-06}, {-0.0008215284708500001, "Field Reading"=9.96679152334026e-06}, {-0.0008217407858999999, "Field Reading"=1.0026902610564895e-05}, {-0.0008276328146499999, "Field Reading"=9.844423938961241e-06}, {-0.00083345962125, "Field Reading"=9.892476299881349e-06}, {-0.0008377560497000001, "Field Reading"=9.897212557668268e-06}, {-0.0008491296067999999, "Field Reading"=9.83242825181531e-06}, {-0.0008535548172, "Field Reading"=9.78436188907773e-06}, {-0.0008602954997000001, "Field Reading"=9.780159949903043e-06}, {-0.0008634908043500001, "Field Reading"=9.775588704832127e-06}, {-0.0008663649374500001, "Field Reading"=9.66597190118485e-06}, {-0.0008731592179500001, "Field Reading"=9.746555878450217e-06}, {-0.0008792073969000001, "Field Reading"=9.709086384558608e-06}, {-0.00087882752715, "Field Reading"=9.678702696329836e-06}, {-0.00088570849165, "Field Reading"=9.596805575135188e-06}, {-0.0008864817794500001, "Field Reading"=9.53727995455328e-06}, {-0.0008925269032499999, "Field Reading"=9.558357342876952e-06}, {-0.0008966638338500001, "Field Reading"=9.577120564261706e-06}, {-0.0009016204634500003, "Field Reading"=9.456976714405613e-06}, {-0.0009084058561000001, "Field Reading"=9.490700376770218e-06}, {-0.0009145637935, "Field Reading"=9.526167033904256e-06}, {-0.0009171811661, "Field Reading"=9.452123669049726e-06}, {-0.00094487197115, "Field Reading"=9.43683135745101e-06}, {-0.0009718710058999999, "Field Reading"=9.284608277047465e-06}, {-0.0009974961995999998, "Field Reading"=9.270421286783148e-06}, {-0.0010229655325, "Field Reading"=9.156294683032267e-06}, {-0.001052452734, "Field Reading"=9.10905341655773e-06}, {-0.0010769300805000001, "Field Reading"=9.027250694550671e-06}, {-0.0011057502780000002, "Field Reading"=9.100066972043792e-06}, {-0.0011358273555000002, "Field Reading"=9.096477820519693e-06}, {-0.0011610196529999999, "Field Reading"=8.969890563875718e-06}, {-0.0011867192995, "Field Reading"=8.971534370429619e-06}, {-0.001215968091, "Field Reading"=9.03906172192829e-06}, {-0.0012451501894999999, "Field Reading"=8.939041425751918e-06}, {-0.001280414172, "Field Reading"=8.904846526915873e-06}, {-0.001301874571, "Field Reading"=8.916296257879076e-06}, {-0.0013296938729999998, "Field Reading"=8.947726711256585e-06}, {-0.0013569264919999998, "Field Reading"=8.85016016966443e-06}, {-0.0013868245955000003, "Field Reading"=8.838554309919458e-06}, {-0.0014156738410000002, "Field Reading"=8.992480538417717e-06}, {-0.001439544324, "Field Reading"=8.85595028782889e-06}, {-0.0014683081220000001, "Field Reading"=8.813095557835579e-06}, {-0.0014955474789999999, "Field Reading"=8.86782348829236e-06}, {-0.0015272694825000002, "Field Reading"=8.934829225787595e-06}, {-0.0015604565005000002, "Field Reading"=8.760392702370496e-06}, {-0.001586399622, "Field Reading"=8.80721331283997e-06}, {-0.0016130595005000002, "Field Reading"=8.873939354100682e-06}, {-0.0016438354175000002, "Field Reading"=8.893752805673661e-06}, {-0.0016710378799999997, "Field Reading"=8.785756150077331e-06}, {-0.0016986270980000003, "Field Reading"=8.798230843512233e-06}, {-0.0017309022369999996, "Field Reading"=8.935252567058772e-06}, {-0.0017606270430000001, "Field Reading"=8.763694805648187e-06}, {-0.0017875542260000002, "Field Reading"=8.712532535438561e-06}, {-0.0018179781695000004, "Field Reading"=8.918430646213751e-06}, {-0.0018456515680000004, "Field Reading"=8.866381485907792e-06}, {-0.0018729793535, "Field Reading"=8.67357571367737e-06}, {-0.0018963426125000002, "Field Reading"=8.811464926975151e-06}, {-0.0019262222059999996, "Field Reading"=8.958341890253187e-06}, {-0.0019524740959999999, "Field Reading"=8.767790433875556e-06}, {-0.0019808823515, "Field Reading"=8.743473613736861e-06}]
  out "DC Voltage (V) 2":dbl=-0.0019808823515
  out "dI/dV (ohm) 2":dbl=8.743473613736861e-06
  out "dV (V) 2":dbl=8.223089583294991e-06
  out "dI (A) 2":dbl=7.18983667949342e-11
  in  "DC Voltage averaging 2":dbl=20.0 format="%#_13g"
  out "Vset (V) 2":dbl=-0.30000000000000016
  in  "MFLI Averaging (Device2)":dbl=100.0 format="%#_13g"
  out "File path 2":path=path "D:/Pranava/Data/STS/MA2158 new mask/012_MA2158_STS_[Dev150]_baseT_2T(89.25deg)_measureX_40uV_17.7777Hz_ground_100xaverage_finescan.dat"
  in  "DC Current Limit (A)":dbl=0.0001 format="%#_13g"
  in  "Keithley 2636B (channel A and B)":refnum<visa-resource-name>="GPIB0::26::INSTR"
  in  "stop":bool
  out "Time (s)":dbl=5682.703
  in  "Folder":path=path "D:/Pranava/Data/STS/MA2158 new mask"
  out "data":dbl[](array[numeric])=[5682.703, 0.0014786366844999998, 2.35323775186076e-11, 9.558138228782806e-06, 2.4620252349713466e-06, -0.30000000000000016, -3.0000000000000016e-09]
  out "File path 1":path=path "D:/Pranava/Data/STS/MA2158 new mask/011_MA2158_STS_[Dev90]_baseT_2T(89.25deg)_measureX_40uV_7.919Hz_ground_100xaverage_finescan.dat"
  # ".dat"
  # "Set Voltage sweep Device 1 (V)"
  # ".dat"
  # "Set Voltage sweep Device 2 (V)"
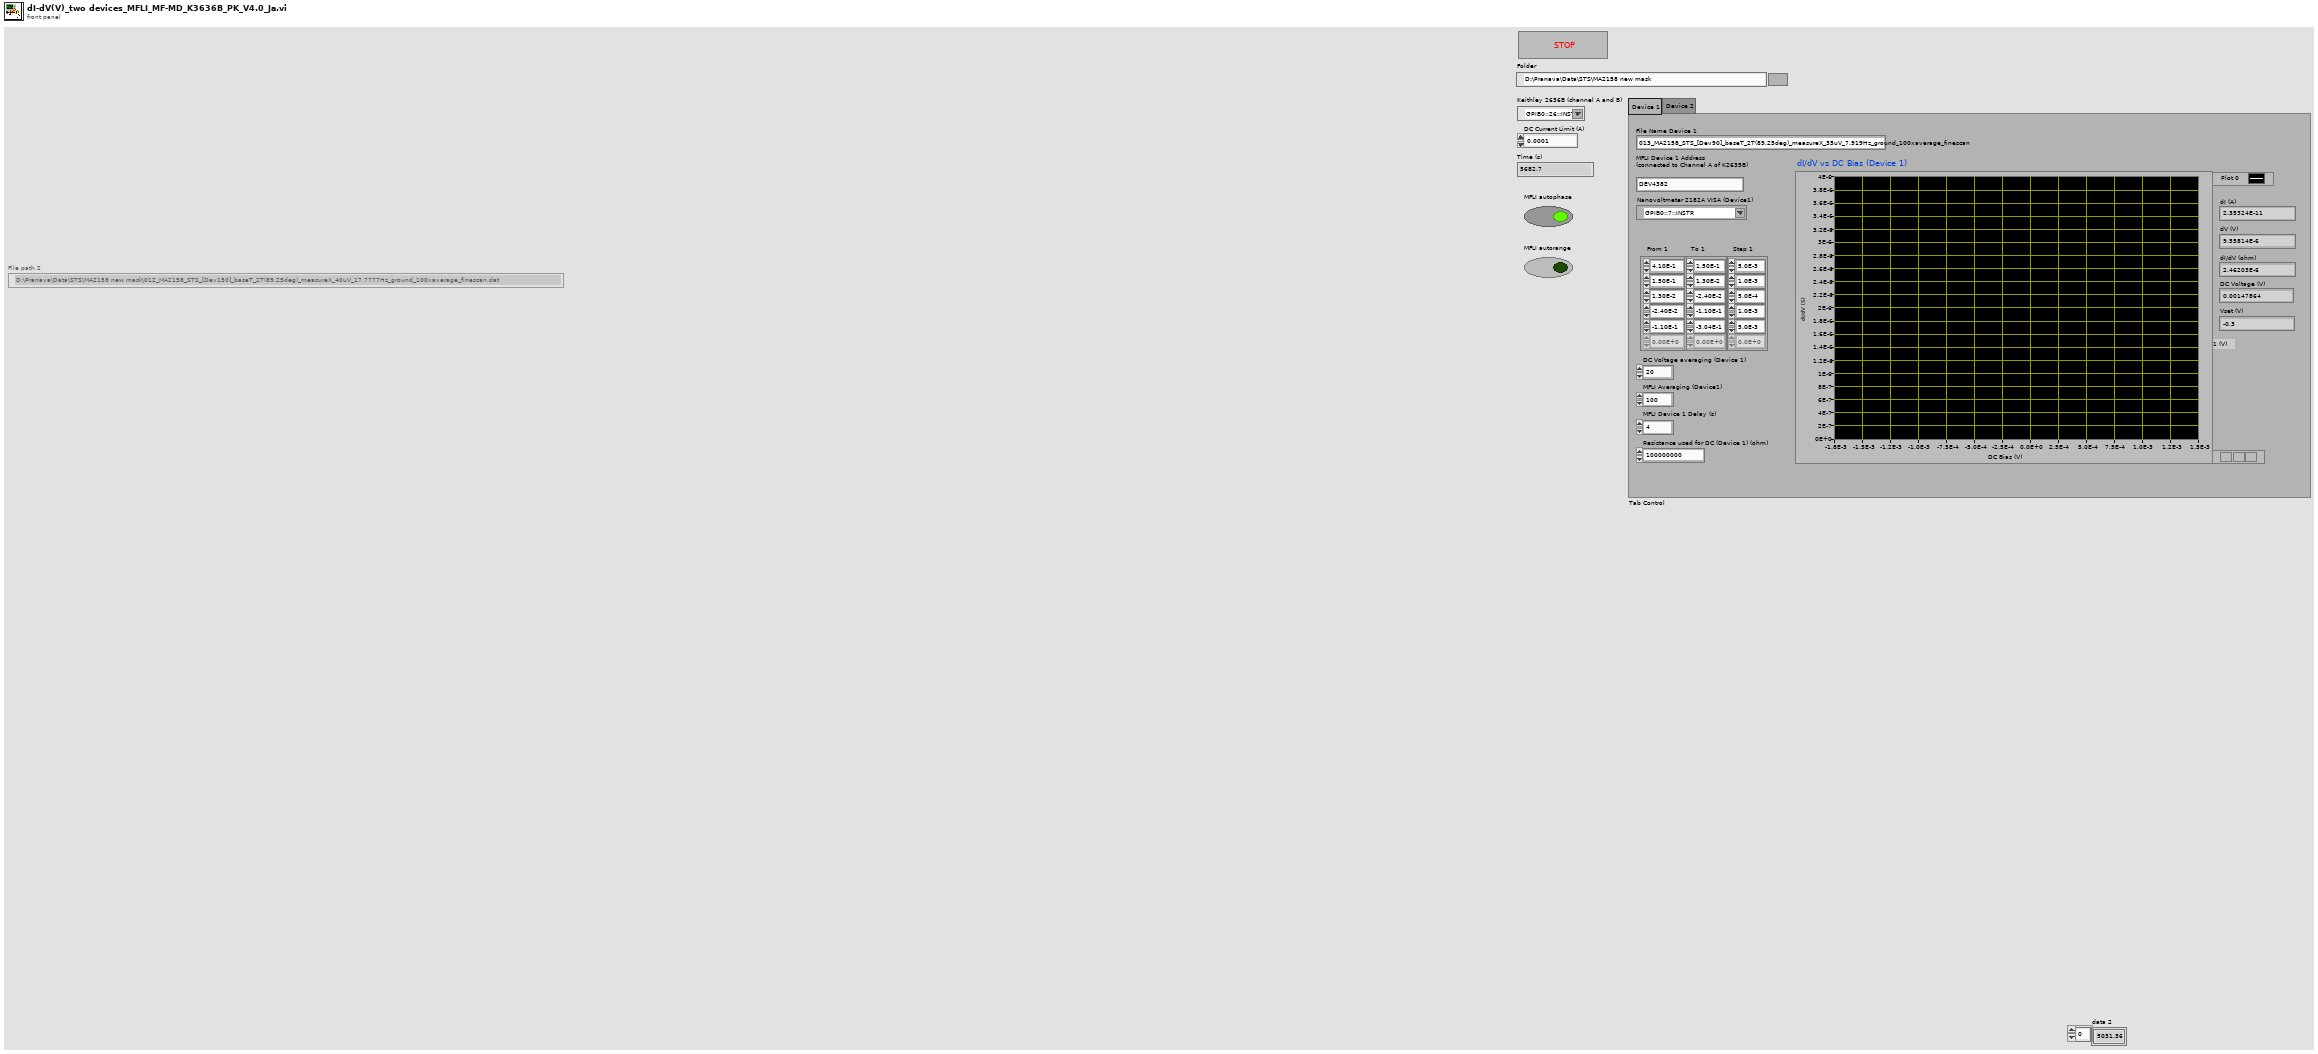
[diagram p1: front panel]
types:
  T1 = enum16{"open", "replace", "create", "open or create", "replace or create", "replace or create with confirmation"}
  T2 = typedef "Zurich Instruments LabOne.lvlib/ziTypeHandle.ctl" = cluster{"handleValid":bool, "Conn":u64, "Path Prefix":string, "Handle":u64, "Connected":bool, "Clockbase(s)":dbl}
  T3 = typedef "Zurich Instruments LabOne.lvlib/ziTypeDemodSampleSingle.ctl" = cluster{"Timestamps (ticks)":u64, "X (Vrms)":dbl, "Y (Vrms)":dbl, "Osc Phase (deg)":dbl, "Freq (Hz)":dbl, "DIO":u32, "AuxIn0 (V)":dbl, "AuxIn1 (V)":dbl, "Trigger":u32}
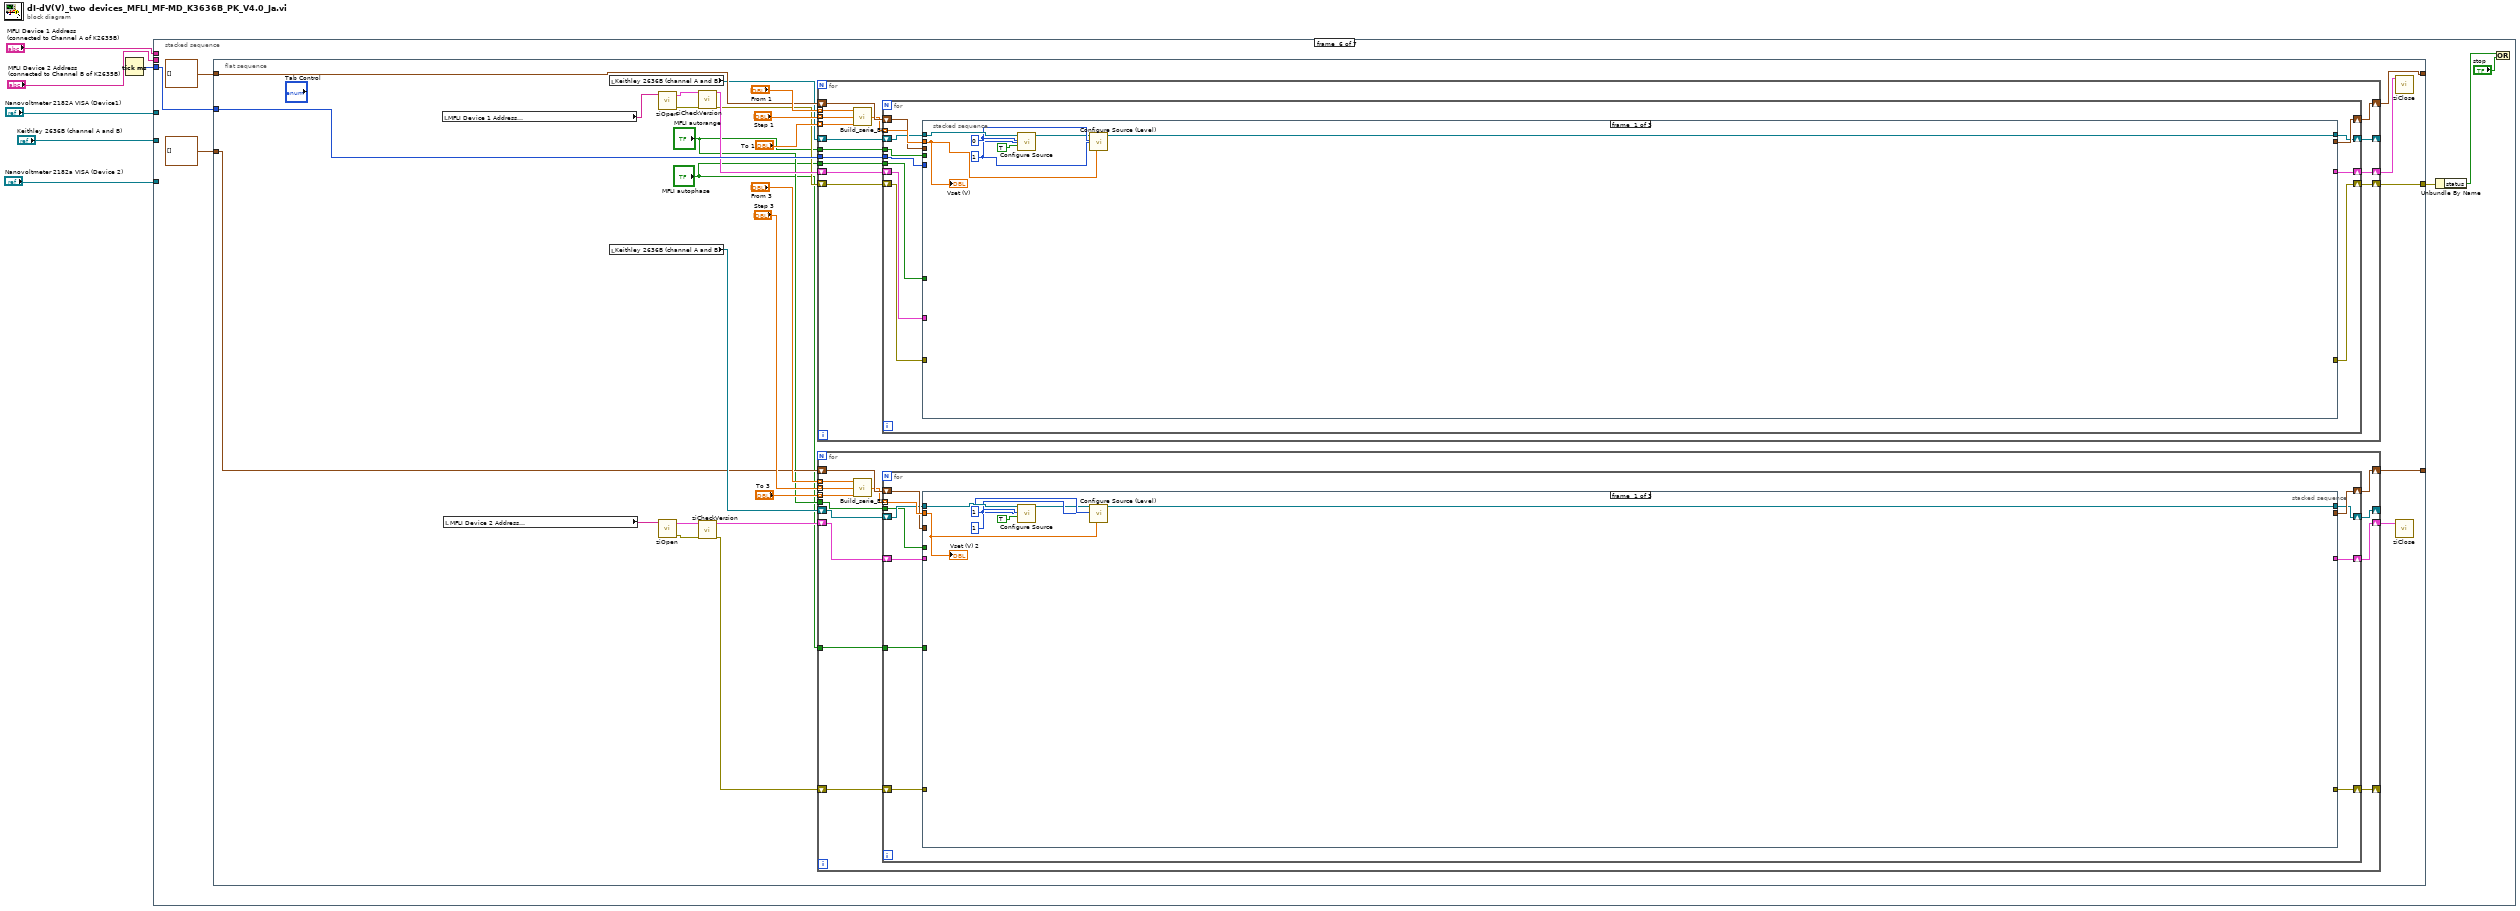
[diagram p0: block diagram]
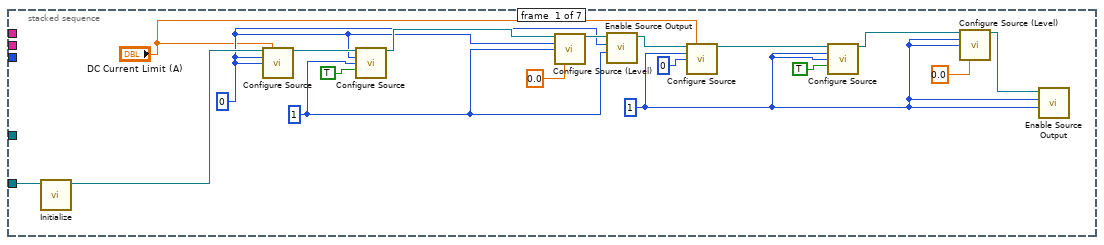
[diagram p2: hidden frame]
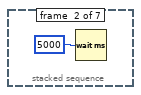
[diagram p3: hidden frame]
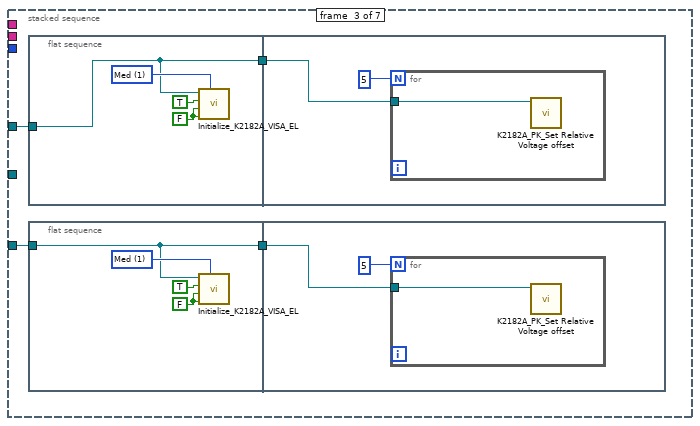
[diagram p4: hidden frame]
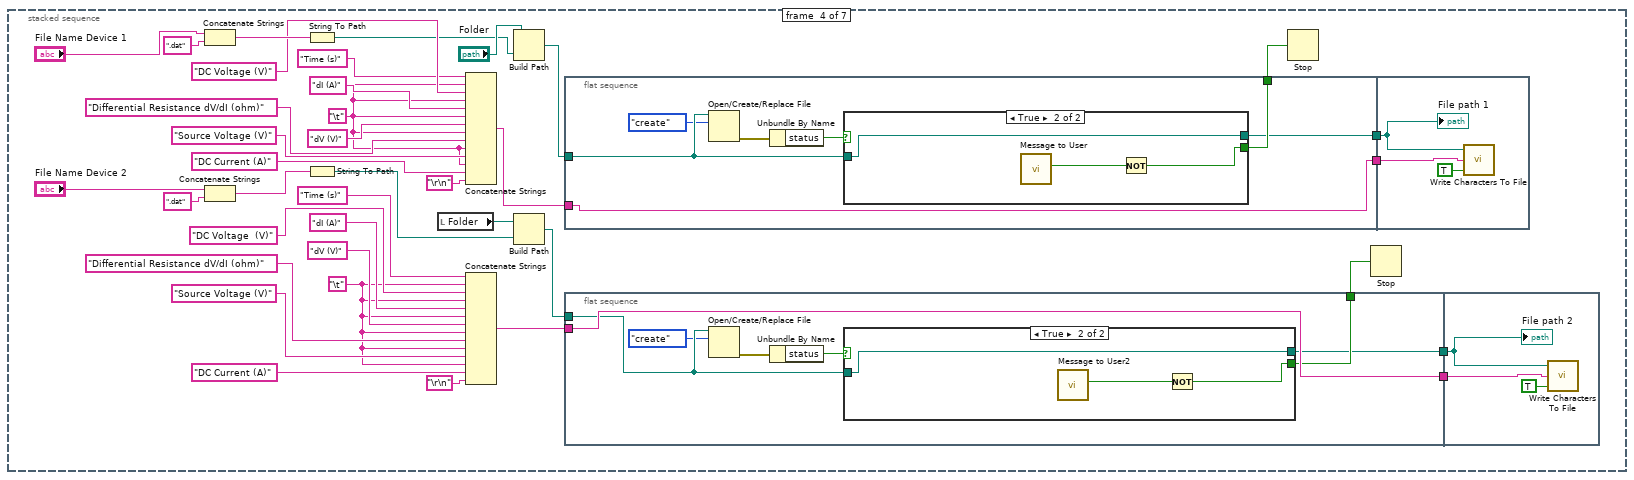
[diagram p5: hidden frame]
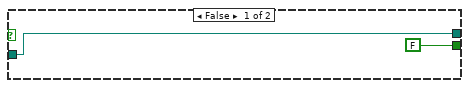
[diagram p6: hidden frame]
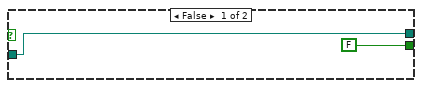
[diagram p7: hidden frame]
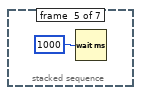
[diagram p8: hidden frame]
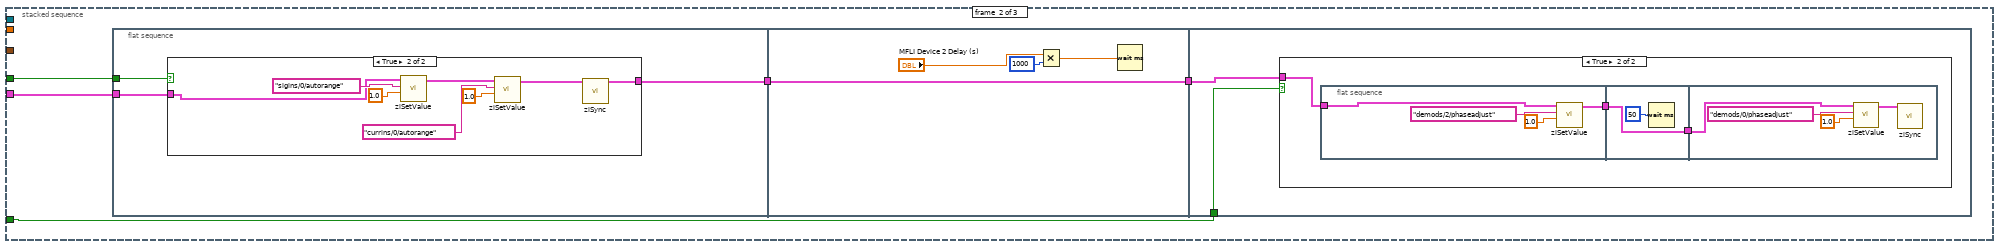
[diagram p9: hidden frame]
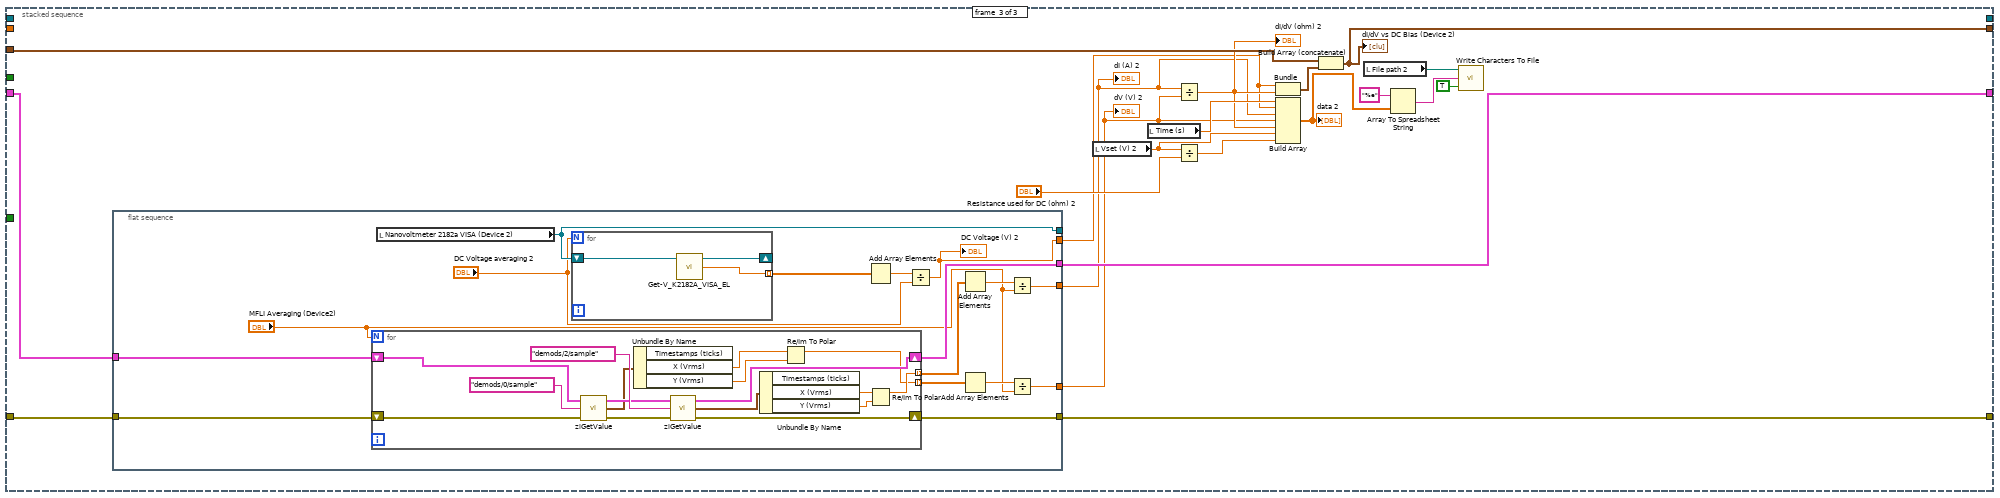
[diagram p12: hidden frame]
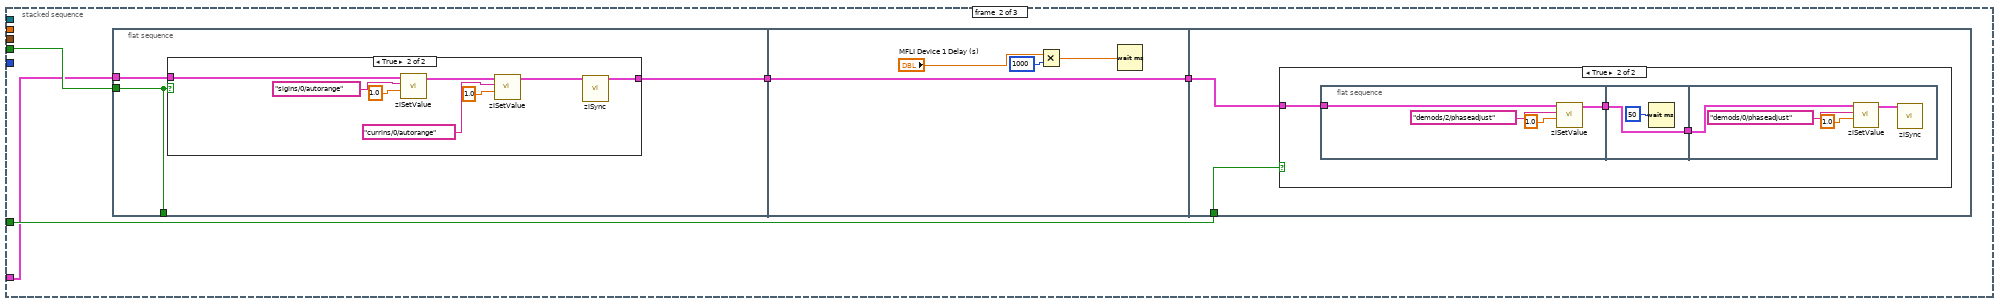
[diagram p13: hidden frame]
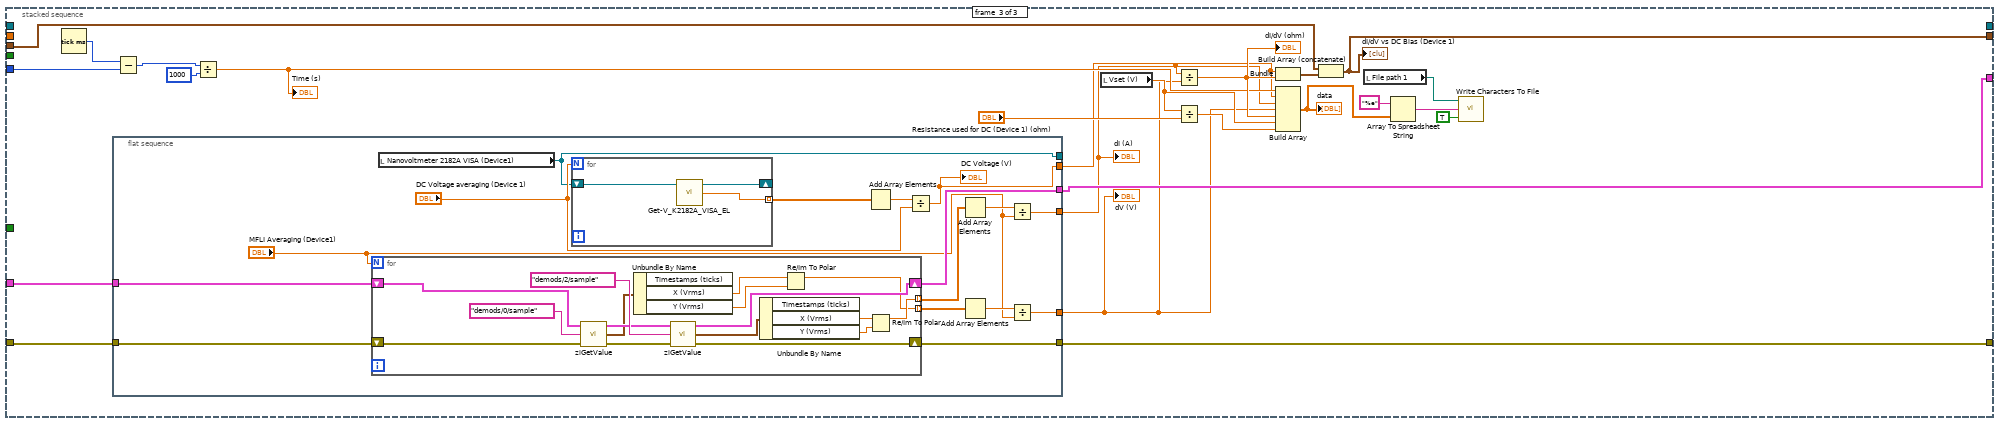
[diagram p16: hidden frame]
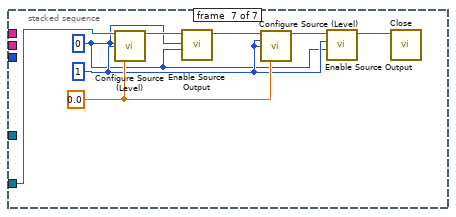
[diagram p17: hidden frame]
diagram:
  n1 = Tick Count (ms)() -> (millisecond timer value=w4:u32)
  n2 = stacked-sequence {
    tunnel: "Nanovoltmeter 2182A VISA (Device1)" -> [_ _ w29 _ _ _ _]
    tunnel: "MFLI Device 1 Address\n(connected to Channel A of K2635B)" -> [_ _ _ _ _ _ _]
    tunnel: w4 -> [_ _ _ _ _ w117 _]
    tunnel: "Keithley 2636B (channel A and B)" -> [w24 _ _ _ _ _ w405]
    tunnel: "Nanovoltmeter 2182a VISA (Device 2)" -> [_ _ w26 _ _ _ _]
    tunnel: "MFLI Device 2 Address\n(connected to Channel B of K2635B)" -> [_ _ _ _ _ _ _]
    frame #0 {
      w7 = 1
      w18 = 0
      w16 = 1
      n3 = call <instrlib>:"Initialize.vi"("VISA resource name"=w24) -> ("VISA resource name out"=w23:refnum<visa-resource-name>)  [unwired: 9 in, 1 out]
      n4 = call-poly <instrlib>:"Configure Source.vi"("VISA resource name"=w23, "Current Limit (0.1 A)"="DC Current Limit (A)", "Source Measure Unit Channel (0: Channel A)"=w18, "Limit Type (1: Voltage)"=w18) -> ("VISA resource name out"=w22:refnum<visa-resource-name>)  [unwired: 10 in, 1 out]
      n5 = call-poly <instrlib>:"Configure Source.vi"("VISA resource name"=w22, "Source Measure Unit Channel (0: Channel A)"=w18, "Range Type (1: Voltage)"=w16, "Auto Range (T: Enable)"=TRUE) -> ("VISA resource name out"=w21:refnum<visa-resource-name>)  [unwired: 10 in, 1 out]
      n6 = call <instrlib>:"Configure Source (Level).vi"("VISA resource name"=w21, "Source Measure Unit Channel (0: Channel A)"=w18, "Level Type (1: Voltage)"=w16, "Voltage Level (0 V)"=0.0) -> ("VISA resource name out"=w20:refnum<visa-resource-name>)  [unwired: 10 in, 1 out]
      n7 = call <instrlib>:"Enable Source Output.vi"("Output Mode (0: Turn off)"=w16, "Source Measure Unit Channel (0: Channel A)"=w18, "VISA resource name"=w20) -> ("VISA resource name out"=w10:refnum<visa-resource-name>)  [unwired: 7 in, 1 out]
      n8 = call-poly <instrlib>:"Configure Source.vi"("VISA resource name"=w10, "Current Limit (0.1 A)"="DC Current Limit (A)", "Source Measure Unit Channel (0: Channel A)"=w7, "Limit Type (1: Voltage)"=0) -> ("VISA resource name out"=w15:refnum<visa-resource-name>)  [unwired: 10 in, 1 out]
      n9 = call-poly <instrlib>:"Configure Source.vi"("VISA resource name"=w15, "Source Measure Unit Channel (0: Channel A)"=w7, "Range Type (1: Voltage)"=w7, "Auto Range (T: Enable)"=TRUE) -> ("VISA resource name out"=w14:refnum<visa-resource-name>)  [unwired: 10 in, 1 out]
      n10 = call <instrlib>:"Configure Source (Level).vi"("VISA resource name"=w14, "Source Measure Unit Channel (0: Channel A)"=w7, "Level Type (1: Voltage)"=w7, "Voltage Level (0 V)"=0.0) -> ("VISA resource name out"=w13:refnum<visa-resource-name>)  [unwired: 10 in, 1 out]
      n11 = call <instrlib>:"Enable Source Output.vi"("Output Mode (0: Turn off)"=w7, "Source Measure Unit Channel (0: Channel A)"=w7, "VISA resource name"=w13) -> ()  [unwired: 7 in, 2 out]
    }
    frame #1 {
      n12 = Wait (ms)(milliseconds to wait=5000) -> ()  [unwired: 1 out]
    }
    frame #2 {
      n13 = flat-sequence {
        tunnel: w29 -> [w37]
        tunnel: [w37] -> w28
        tunnel: w28 -> [w41]
        frame #0 {
          w39 = u16 1 items=["Slow", "Med", "Fast"] ("Rate (NPLC)")
          w40 = FALSE ("Auto range?")
          n14 = call "Initialize_K2182A_VISA_EL.vi"("VISA address"=w37, "Auto range?"=TRUE, "Analog LPass\nFilter?"=w40, "DC\nFilter?"=w40, "Rate (NPLC)"=w39) -> ()  [unwired: 1 in, 1 out]
        }
        frame #1 {
          n15 = for {
            N: 5 ("Numeric") -> [_]
            tunnel: w41 -> [w43]
            n16 = call "K2182A_PK_Set Relative Voltage offset.vi"("VISA address"=w43) -> ()  [unwired: 11 in]
          }
        }
      }
      n17 = flat-sequence {
        tunnel: w26 -> [w30]
        tunnel: [w30] -> w27
        tunnel: w27 -> [w34]
        frame #0 {
          w32 = u16 1 items=["Slow", "Med", "Fast"] ("Rate (NPLC)")
          w33 = FALSE ("Auto range?")
          n18 = call "Initialize_K2182A_VISA_EL.vi"("VISA address"=w30, "Auto range?"=TRUE, "Analog LPass\nFilter?"=w33, "DC\nFilter?"=w33, "Rate (NPLC)"=w32) -> ()  [unwired: 1 in, 1 out]
        }
        frame #1 {
          n19 = for {
            N: 5 ("Numeric") -> [_]
            tunnel: w34 -> [w36]
            n20 = call "K2182A_PK_Set Relative Voltage offset.vi"("VISA address"=w36) -> ()  [unwired: 11 in]
          }
        }
      }
    }
    frame #3 {
      w47 = "\t"
      w64 = "\t"
      n21 = Concatenate Strings("File Name Device 1", ".dat" ("string")) -> (w78:string)
      n22 = Concatenate Strings("File Name Device 2", ".dat" ("string")) -> (w59:string)
      n23 = String To Path(string=w78) -> (path=w70:path)
      n24 = String To Path(string=w59) -> (path=w53:path)
      n25 = local read "Folder"() -> (w45:path)
      n26 = Concatenate Strings("Time (s)", w64, "DC Voltage (V)" ("string"), w64, "dI (A)" ("string"), w64, "dV (V)" ("string"), w64, "Differential Resistance dV/dI (ohm)", w64, "Source Voltage (V)", w64, "DC Current (A)", "\r\n") -> (w79:string)
      n27 = Concatenate Strings("Time (s)", w47, "DC Voltage  (V)" ("string"), w47, "dI (A)" ("string"), w47, "dV (V)" ("string"), w47, "Differential Resistance dV/dI (ohm)", w47, "Source Voltage (V)", w47, "DC Current (A)", "\r\n") -> (w60:string)
      n28 = Build Path(base path="Folder", name or relative path=w70) -> (appended path=w69:path)
      n29 = Build Path(base path=w45, name or relative path=w53) -> (appended path=w52:path)
      n30 = flat-sequence {
        tunnel: w69 -> [w100]
        tunnel: w79 -> [w103]
        tunnel: [w103] -> w81
        tunnel: [w102] -> w76
        tunnel: [w101] -> w80
        tunnel: w81 -> [w110]
        tunnel: w80 -> [w109]
        frame #0 {
          n31 = Open/Create/Replace File(file path (use dialog)=w100, operation (0:open)=T1."create") -> (error out=w99:errorcluster)  [unwired: 4 in, 2 out]
          n32 = Unbundle By Name(w99) -> ("status"=w97:bool)
          n33 = case shown="True" w97 {
            tunnel: [FALSE ("Yes") w107] -> w102
            tunnel: [w104 w106] -> w101
            tunnel: w100 -> [w104 w106]
            frame False {
            }
            frame True {
              n34 = call "Message to User"() -> ("Yes"=w108:bool)  [unwired: 10 in, 1 out]
              n35 = Not(x=w108) -> (.not. x?=w107:bool)
            }
          }
        }
        frame #1 {
          n36 = call <vilib>:"Write Characters To File.vi"("append to file? (new file:F)"=TRUE, "character string"=w110, "file path (dialog if empty)"=w109) -> ()  [unwired: 2 in, 1 out]
          "File path 1" <- w109
        }
      }
      n37 = flat-sequence {
        tunnel: w52 -> [w85]
        tunnel: w60 -> [w88]
        tunnel: [w88] -> w62
        tunnel: [w87] -> w58
        tunnel: [w86] -> w61
        tunnel: w62 -> [w95]
        tunnel: w61 -> [w94]
        frame #0 {
          n38 = Open/Create/Replace File(file path (use dialog)=w85, operation (0:open)=T1."create") -> (error out=w84:errorcluster)  [unwired: 4 in, 2 out]
          n39 = Unbundle By Name(w84) -> ("status"=w82:bool)
          n40 = case shown="True" w82 {
            tunnel: [FALSE ("Yes") w92] -> w87
            tunnel: [w89 w91] -> w86
            tunnel: w85 -> [w89 w91]
            frame False {
            }
            frame True {
              n41 = call "Message to User2"() -> ("Yes"=w93:bool)  [unwired: 10 in, 1 out]
              n42 = Not(x=w93) -> (.not. x?=w92:bool)
            }
          }
        }
        frame #1 {
          n43 = call <vilib>:"Write Characters To File.vi"("append to file? (new file:F)"=TRUE, "character string"=w95, "file path (dialog if empty)"=w94) -> ()  [unwired: 2 in, 1 out]
          "File path 2" <- w94
        }
      }
      n44 = Stop(stop? (T)=w76) -> ()
      n45 = Stop(stop? (T)=w58) -> ()
    }
    frame #4 {
      n46 = Wait (ms)(milliseconds to wait=u32 1000) -> ()  [unwired: 1 out]
    }
    frame #5 {
      n47 = flat-sequence {
        tunnel: [w141] -> w115
        tunnel: [w140] -> _
        tunnel: [w125] -> _
        tunnel: cluster{dbl, "Field Reading":dbl}[] [] -> [w121]
        tunnel: cluster{dbl, "Field Reading":dbl}[] [] -> [w143]
        tunnel: w117 -> [w142]
        frame #0 {
          n48 = local read "MFLI Device 1 Address\n(connected to Channel A of K2635B)"() -> (w137:string)
          n49 = local read "MFLI Device 2 Address\n(connected to Channel B of K2635B)"() -> (w130:string)
          n50 = local read "Keithley 2636B (channel A and B)"() -> (w133:refnum<visa-resource-name>)
          n51 = local read "Keithley 2636B (channel A and B)"() -> (w126:refnum<visa-resource-name>)
          n52 = call <instrlib>:"ziOpen.vi"("Address"=w137) -> ("Error Out"=w136:errorcluster, "HandleOut"=w139:T2)  [unwired: 3 in, 1 out]
          n53 = call <instrlib>:"ziOpen.vi"("Address"=w130) -> ("Error Out"=w129:errorcluster, "HandleOut"=w132:T2)  [unwired: 3 in, 1 out]
          n54 = call <instrlib>:"ziCheckVersion.vi"("Handle In"=w139, "Error In"=w136) -> ("Handle Out"=w138:T2, "Error Out"=w135:errorcluster)  [unwired: 11 in, 1 out]
          n55 = call <instrlib>:"ziCheckVersion.vi"("Handle In"=w132, "Error In"=w129) -> ("Handle Out"=w131:T2, "Error Out"=w128:errorcluster)  [unwired: 11 in, 1 out]
          n56 = for {
            tunnel: "From 1" -> [w281] mode=indexing
            tunnel: "To 1" -> [w280] mode=indexing
            tunnel: "Step 1" -> [w279] mode=indexing
            shift-right: [w283] -> w140
            shift-left: w143 -> [w284]
            tunnel: w142 -> [w278]
            shift-right: [w276] -> w134
            shift-left: w138 -> [w277]
            shift-right: [w275] -> w141
            shift-left: w135 -> [w274]
            shift-right: [w272] -> _
            shift-left: w133 -> [w273]
            tunnel: "MFLI autorange" -> [w271]
            tunnel: "MFLI autophase" -> [w270]
            n57 = call "Build_serie_EL.vi"("end value"=w280, "increment"=w279, "start value"=w281) -> ("output array"=w282:dbl[])
            n58 = for {
              tunnel: w282 -> [w296] mode=indexing
              shift-right: [w294] -> w283
              shift-left: w284 -> [w295]
              tunnel: w278 -> [w293]
              shift-right: [w291] -> w276
              shift-left: w277 -> [w292]
              shift-right: [w290] -> w275
              shift-left: w274 -> [w289]
              shift-right: [w287] -> w272
              shift-left: w273 -> [w288]
              tunnel: w271 -> [w286]
              tunnel: w270 -> [w285]
              n59 = stacked-sequence {
                tunnel: w295 -> [_ _ w362]
                tunnel: w296 -> [w303 _ _]
                tunnel: [_ _ w361] -> w294
                tunnel: w293 -> [_ _ w358]
                tunnel: w292 -> [_ w304 w354]
                tunnel: [_ _ w353] -> w291
                tunnel: [_ _ w352] -> w290
                tunnel: w289 -> [_ _ w351]
                tunnel: w288 -> [w301 _ _]
                tunnel: [w302 _ _] -> w287
                tunnel: w286 -> [_ w306 _]
                tunnel: w285 -> [_ w305 _]
                frame #0 {
                  w300 = 0
                  w299 = 1
                  n60 = call-poly <instrlib>:"Configure Source.vi"("VISA resource name"=w301, "Source Measure Unit Channel (0: Channel A)"=w300, "Range Type (1: Voltage)"=w299, "Auto Range (T: Enable)"=TRUE) -> ("VISA resource name out"=w297:refnum<visa-resource-name>)  [unwired: 10 in, 1 out]
                  n61 = call <instrlib>:"Configure Source (Level).vi"("VISA resource name"=w297, "Source Measure Unit Channel (0: Channel A)"=w300, "Level Type (1: Voltage)"=w299, "Voltage Level (0 V)"=w303) -> ("VISA resource name out"=w302:refnum<visa-resource-name>)  [unwired: 10 in, 1 out]
                  "Vset (V)" <- w303
                }
                frame #1 {
                  n62 = flat-sequence {
                    tunnel: [w309] -> _
                    tunnel: w304 -> [w311]
                    tunnel: [w310] -> w308
                    tunnel: w306 -> [w309]
                    tunnel: [w321] -> w307
                    tunnel: w308 -> [w321]
                    tunnel: w307 -> [w326]
                    tunnel: w305 -> [w325]
                    frame #0 {
                      n63 = case shown="True" w309 {
                        tunnel: w311 -> [w312 w314]
                        tunnel: [w312 w313] -> w310
                        frame False {
                        }
                        frame True {
                          n64 = call-poly <instrlib>:"ziSetValue.vi"("Value"=1.0, "Path"="sigins/0/autorange", "Handle In"=w314) -> ("Handle Out"=w319:T2)  [unwired: 2 in, 1 out]
                          n65 = call-poly <instrlib>:"ziSetValue.vi"("Value"=1.0, "Path"="currins/0/autorange", "Handle In"=w319) -> ("Handle Out"=w320:T2)  [unwired: 2 in, 1 out]
                          n66 = call <instrlib>:"ziSync.vi"("Handle In"=w320) -> ("Handle Out"=w313:T2)  [unwired: 13 in, 1 out]
                        }
                      }
                    }
                    frame #1 {
                      n67 = Multiply(x="MFLI Device 1 Delay (s)", y=1000) -> (x*y=w324:dbl)
                      n68 = Wait (ms)(milliseconds to wait=w324) -> ()  [unwired: 1 out]
                    }
                    frame #2 {
                      n69 = case shown="True" w325 {
                        tunnel: w326 -> [_ w327]
                        frame False {
                        }
                        frame True {
                          n70 = flat-sequence {
                            tunnel: [w333] -> w329
                            tunnel: w327 -> [w330]
                            tunnel: w329 -> [w335]
                            tunnel: [w335] -> w328
                            tunnel: w328 -> [w336]
                            frame #0 {
                              n71 = call-poly <instrlib>:"ziSetValue.vi"("Value"=1.0, "Path"="demods/2/phaseadjust", "Handle In"=w330) -> ("Handle Out"=w333:T2)  [unwired: 2 in, 1 out]
                            }
                            frame #1 {
                              n72 = Wait (ms)(milliseconds to wait=50) -> ()  [unwired: 1 out]
                            }
                            frame #2 {
                              n73 = call-poly <instrlib>:"ziSetValue.vi"("Value"=1.0, "Path"="demods/0/phaseadjust", "Handle In"=w336) -> ("Handle Out"=w337:T2)  [unwired: 2 in, 1 out]
                              n74 = call <instrlib>:"ziSync.vi"("Handle In"=w337) -> ()  [unwired: 13 in, 2 out]
                            }
                          }
                        }
                      }
                    }
                  }
                }
                frame #2 {
                  n75 = Tick Count (ms)() -> (millisecond timer value=w359:u32)
                  n76 = flat-sequence {
                    tunnel: [w369] -> w342
                    tunnel: [w367] -> w341
                    tunnel: [w378] -> w352
                    tunnel: [w379] -> w353
                    tunnel: [w374] -> _
                    tunnel: w351 -> [w372]
                    tunnel: w354 -> [w373]
                    tunnel: [w364] -> w340
                    frame #0 {
                      n77 = for {
                        N: "MFLI Averaging (Device1)" -> [_]
                        tunnel: [w393] -> w366 mode=indexing
                        tunnel: [w392] -> w368 mode=indexing
                        shift-right: [w395] -> w379
                        shift-left: w373 -> [w381]
                        shift-right: [w394] -> w378
                        shift-left: w372 -> [w380]
                        n78 = call-poly <instrlib>:"ziGetValue.vi"("error in"=w380, "Path"="demods/0/sample", "Handle In"=w381) -> ("error out"=w386:errorcluster, "Demod Sample Out"=w384:T3, "Handle Out"=w387:T2)
                        n79 = Unbundle By Name(w384) -> ("X (Vrms)"=w383:dbl, "Y (Vrms)"=w382:dbl)  [unwired: 1 out]
                        n80 = call-poly <instrlib>:"ziGetValue.vi"("error in"=w386, "Path"="demods/2/sample", "Handle In"=w387) -> ("error out"=w394:errorcluster, "Demod Sample Out"=w390:T3, "Handle Out"=w395:T2)
                        n81 = Unbundle By Name(w390) -> ("X (Vrms)"=w389:dbl, "Y (Vrms)"=w388:dbl)  [unwired: 1 out]
                        n82 = Re/Im To Polar(2:w382, 3:w383) -> (1:w392:dbl)  [unwired: 1 out]
                        n83 = Re/Im To Polar(2:w388, 3:w389) -> (1:w393:dbl)  [unwired: 1 out]
                      }
                      n84 = local read "Nanovoltmeter 2182A VISA (Device1)"() -> (w374:refnum<visa-resource-name>)
                      n85 = for {
                        N: "DC Voltage averaging (Device 1)" -> [_]
                        tunnel: [w397] -> w376 mode=indexing
                        shift-right: [w396] -> _
                        shift-left: w374 -> [w398]
                        n86 = call "Get-V_K2182A_VISA_EL.vi"("VISA K2182A"=w398) -> ("V (V)"=w397:dbl, "VISA K2182A"=w396:refnum<visa-resource-name>)  [unwired: 2 in, 1 out]
                      }
                      n87 = Add Array Elements(numeric array=w376) -> (sum=w377:dbl)
                      n88 = Divide(x=w377, y="DC Voltage averaging (Device 1)") -> (x/y=w364:dbl)
                      "DC Voltage (V)" <- w364
                      n89 = Add Array Elements(numeric array=w366) -> (sum=w371:dbl)
                      n90 = Add Array Elements(numeric array=w368) -> (sum=w370:dbl)
                      n91 = Divide(x=w371, y="MFLI Averaging (Device1)") -> (x/y=w367:dbl)
                      n92 = Divide(x=w370, y="MFLI Averaging (Device1)") -> (x/y=w369:dbl)
                    }
                  }
                  n93 = Subtract(x=w359, y=w358) -> (x-y=w357:u32)
                  n94 = Divide(x=w357, y=1000) -> (x/y=w355:dbl)
                  "Time (s)" <- w355
                  n95 = local read "Vset (V)"() -> (w344:dbl)
                  n96 = Divide(x=w341, y=w342) -> (x/y=w360:dbl)
                  "dI/dV (ohm)" <- w360
                  n97 = Divide(x=w344, y="Resistance used for DC (Device 1) (ohm)") -> (x/y=w343:dbl)
                  n98 = Bundle(w340, w360) -> (w363:cluster{dbl, dbl})  [unwired: 1 in]
                  n99 = Build Array(w355, w340, w341, w342, w360, w344, w343) -> (w346:dbl[])
                  "data" <- w346
                  n100 = Build Array (concatenate)(w362, w363) -> (w361:cluster{dbl, "Field Reading":dbl}[])
                  "dI/dV vs DC Bias (Device 1)" <- w361
                  n101 = local read "File path 1"() -> (w348:path)
                  n102 = Array To Spreadsheet String(array=w346, 3:"%e" ("format string")) -> (spreadsheet string=w349:string)  [unwired: 1 in]
                  n103 = call <vilib>:"Write Characters To File.vi"("append to file? (new file:F)"=TRUE, "character string"=w349, "file path (dialog if empty)"=w348) -> ()  [unwired: 2 in, 1 out]
                  "dI (A)" <- w341
                  "dV (V)" <- w342
                }
              }
            }
          }
          n104 = for {
            tunnel: "From 3" -> [w157] mode=indexing
            tunnel: "To 3" -> [w156] mode=indexing
            tunnel: "Step 3" -> [w155] mode=indexing
            shift-right: [w159] -> w125
            shift-left: w121 -> [w160]
            shift-right: [w153] -> w127
            shift-left: w131 -> [w154]
            shift-right: [w152] -> _
            shift-left: w128 -> [w151]
            shift-right: [w149] -> _
            shift-left: w126 -> [w150]
            tunnel: "MFLI autophase" -> [w148]
            tunnel: "MFLI autorange" -> [w147]
            n105 = call "Build_serie_EL.vi"("end value"=w156, "increment"=w155, "start value"=w157) -> ("output array"=w158:dbl[])
            n106 = for {
              tunnel: w158 -> [w171] mode=indexing
              shift-right: [w169] -> w159
              shift-left: w160 -> [w170]
              shift-right: [w167] -> w153
              shift-left: w154 -> [w168]
              shift-right: [w166] -> w152
              shift-left: w151 -> [w165]
              shift-right: [w163] -> w149
              shift-left: w150 -> [w164]
              tunnel: w148 -> [w162]
              tunnel: w147 -> [w161]
              n107 = stacked-sequence {
                tunnel: w170 -> [_ _ w233]
                tunnel: w171 -> [w172 _ _]
                tunnel: [_ _ w218] -> w169
                tunnel: w168 -> [_ w181 w232]
                tunnel: [_ _ w231] -> w167
                tunnel: [_ _ w230] -> w166
                tunnel: w165 -> [_ _ w229]
                tunnel: w164 -> [w177 _ _]
                tunnel: [w178 _ _] -> w163
                tunnel: w162 -> [_ w183 _]
                tunnel: w161 -> [_ w182 _]
                frame #0 {
                  w176 = 1
                  w175 = 1
                  n108 = call-poly <instrlib>:"Configure Source.vi"("VISA resource name"=w177, "Source Measure Unit Channel (0: Channel A)"=w176, "Range Type (1: Voltage)"=w175, "Auto Range (T: Enable)"=TRUE) -> ("VISA resource name out"=w173:refnum<visa-resource-name>)  [unwired: 10 in, 1 out]
                  n109 = call <instrlib>:"Configure Source (Level).vi"("VISA resource name"=w173, "Source Measure Unit Channel (0: Channel A)"=w176, "Level Type (1: Voltage)"=w175, "Voltage Level (0 V)"=w172) -> ("VISA resource name out"=w178:refnum<visa-resource-name>)  [unwired: 10 in, 1 out]
                  "Vset (V) 2" <- w172
                }
                frame #1 {
                  n110 = flat-sequence {
                    tunnel: w182 -> [w186]
                    tunnel: w181 -> [w185]
                    tunnel: [w184] -> w179
                    tunnel: [w196] -> w180
                    tunnel: w179 -> [w196]
                    tunnel: w183 -> [w201]
                    tunnel: w180 -> [w200]
                    frame #0 {
                      n111 = case shown="True" w186 {
                        tunnel: w185 -> [w187 w189]
                        tunnel: [w187 w188] -> w184
                        frame False {
                        }
                        frame True {
                          n112 = call-poly <instrlib>:"ziSetValue.vi"("Value"=1.0, "Path"="sigins/0/autorange", "Handle In"=w189) -> ("Handle Out"=w194:T2)  [unwired: 2 in, 1 out]
                          n113 = call-poly <instrlib>:"ziSetValue.vi"("Value"=1.0, "Path"="currins/0/autorange", "Handle In"=w194) -> ("Handle Out"=w195:T2)  [unwired: 2 in, 1 out]
                          n114 = call <instrlib>:"ziSync.vi"("Handle In"=w195) -> ("Handle Out"=w188:T2)  [unwired: 13 in, 1 out]
                        }
                      }
                    }
                    frame #1 {
                      n115 = Multiply(x="MFLI Device 2 Delay (s)", y=1000) -> (x*y=w199:dbl)
                      n116 = Wait (ms)(milliseconds to wait=w199) -> ()  [unwired: 1 out]
                    }
                    frame #2 {
                      n117 = case shown="True" w201 {
                        tunnel: w200 -> [_ w202]
                        frame False {
                        }
                        frame True {
                          n118 = flat-sequence {
                            tunnel: [w208] -> w204
                            tunnel: w202 -> [w205]
                            tunnel: w204 -> [w210]
                            tunnel: [w210] -> w203
                            tunnel: w203 -> [w211]
                            frame #0 {
                              n119 = call-poly <instrlib>:"ziSetValue.vi"("Value"=1.0, "Path"="demods/2/phaseadjust", "Handle In"=w205) -> ("Handle Out"=w208:T2)  [unwired: 2 in, 1 out]
                            }
                            frame #1 {
                              n120 = Wait (ms)(milliseconds to wait=50) -> ()  [unwired: 1 out]
                            }
                            frame #2 {
                              n121 = call-poly <instrlib>:"ziSetValue.vi"("Value"=1.0, "Path"="demods/0/phaseadjust", "Handle In"=w211) -> ("Handle Out"=w212:T2)  [unwired: 2 in, 1 out]
                              n122 = call <instrlib>:"ziSync.vi"("Handle In"=w212) -> ()  [unwired: 13 in, 2 out]
                            }
                          }
                        }
                      }
                    }
                  }
                }
                frame #2 {
                  n123 = flat-sequence {
                    tunnel: [w239] -> w217
                    tunnel: [w237] -> w216
                    tunnel: [w249] -> w230
                    tunnel: [w250] -> w231
                    tunnel: [w242] -> w215
                    tunnel: [w246] -> _
                    tunnel: w229 -> [w243]
                    tunnel: w232 -> [w244]
                    frame #0 {
                      n124 = for {
                        N: "MFLI Averaging (Device2)" -> [_]
                        tunnel: [w264] -> w236 mode=indexing
                        tunnel: [w263] -> w238 mode=indexing
                        shift-right: [w266] -> w250
                        shift-left: w244 -> [w252]
                        shift-right: [w265] -> w249
                        shift-left: w243 -> [w251]
                        n125 = call-poly <instrlib>:"ziGetValue.vi"("error in"=w251, "Path"="demods/0/sample", "Handle In"=w252) -> ("error out"=w257:errorcluster, "Demod Sample Out"=w255:T3, "Handle Out"=w258:T2)
                        n126 = Unbundle By Name(w255) -> ("X (Vrms)"=w254:dbl, "Y (Vrms)"=w253:dbl)  [unwired: 1 out]
                        n127 = call-poly <instrlib>:"ziGetValue.vi"("error in"=w257, "Path"="demods/2/sample", "Handle In"=w258) -> ("error out"=w265:errorcluster, "Demod Sample Out"=w261:T3, "Handle Out"=w266:T2)
                        n128 = Unbundle By Name(w261) -> ("X (Vrms)"=w260:dbl, "Y (Vrms)"=w259:dbl)  [unwired: 1 out]
                        n129 = Re/Im To Polar(2:w253, 3:w254) -> (1:w263:dbl)  [unwired: 1 out]
                        n130 = Re/Im To Polar(2:w259, 3:w260) -> (1:w264:dbl)  [unwired: 1 out]
                      }
                      n131 = local read "Nanovoltmeter 2182a VISA (Device 2)"() -> (w246:refnum<visa-resource-name>)
                      n132 = for {
                        N: "DC Voltage averaging 2" -> [_]
                        tunnel: [w268] -> w247 mode=indexing
                        shift-right: [w267] -> _
                        shift-left: w246 -> [w269]
                        n133 = call "Get-V_K2182A_VISA_EL.vi"("VISA K2182A"=w269) -> ("V (V)"=w268:dbl, "VISA K2182A"=w267:refnum<visa-resource-name>)  [unwired: 2 in, 1 out]
                      }
                      n134 = Add Array Elements(numeric array=w247) -> (sum=w248:dbl)
                      n135 = Divide(x=w248, y="DC Voltage averaging 2") -> (x/y=w242:dbl)
                      "DC Voltage (V) 2" <- w242
                      n136 = Add Array Elements(numeric array=w236) -> (sum=w240:dbl)
                      n137 = Add Array Elements(numeric array=w238) -> (sum=w241:dbl)
                      n138 = Divide(x=w240, y="MFLI Averaging (Device2)") -> (x/y=w237:dbl)
                      n139 = Divide(x=w241, y="MFLI Averaging (Device2)") -> (x/y=w239:dbl)
                    }
                  }
                  n140 = local read "Vset (V) 2"() -> (w224:dbl)
                  n141 = local read "Time (s)"() -> (w221:dbl)
                  n142 = Divide(x=w216, y=w217) -> (x/y=w219:dbl)
                  "dI/dV (ohm) 2" <- w219
                  n143 = Divide(x=w224, y="Resistance used for DC (ohm) 2") -> (x/y=w223:dbl)
                  n144 = Bundle(w215, w219) -> (w234:cluster{dbl, dbl})  [unwired: 1 in]
                  n145 = Build Array(w221, w215, w216, w217, w219, w224, w223) -> (w222:dbl[])
                  "data 2" <- w222
                  n146 = Build Array (concatenate)(w233, w234) -> (w218:cluster{dbl, "Field Reading":dbl}[])
                  "dI/dV vs DC Bias (Device 2)" <- w218
                  n147 = local read "File path 2"() -> (w226:path)
                  n148 = Array To Spreadsheet String(array=w222, 3:"%e" ("format string")) -> (spreadsheet string=w227:string)  [unwired: 1 in]
                  n149 = call <vilib>:"Write Characters To File.vi"("append to file? (new file:F)"=TRUE, "character string"=w227, "file path (dialog if empty)"=w226) -> ()  [unwired: 2 in, 1 out]
                  "dV (V) 2" <- w217
                  "dI (A) 2" <- w216
                }
              }
            }
          }
          n150 = call <instrlib>:"ziClose.vi"("Handle In"=w134) -> ()  [unwired: 1 in, 4 out]
          n151 = call <instrlib>:"ziClose.vi"("Handle In"=w127) -> ()  [unwired: 1 in, 4 out]
        }
      }
      n152 = Unbundle By Name(w115) -> ("status"=w114:bool)
      n153 = Or(x=w114, y="stop") -> ()  [unwired: 1 out]
    }
    frame #6 {
      w403 = 0.0
      w401 = 0
      w402 = 1
      n154 = call <instrlib>:"Configure Source (Level).vi"("VISA resource name"=w405, "Source Measure Unit Channel (0: Channel A)"=w401, "Level Type (1: Voltage)"=w402, "Voltage Level (0 V)"=w403) -> ("VISA resource name out"=w406:refnum<visa-resource-name>)  [unwired: 10 in, 1 out]
      n155 = call <instrlib>:"Enable Source Output.vi"("Output Mode (0: Turn off)"=w401, "Source Measure Unit Channel (0: Channel A)"=w401, "VISA resource name"=w406) -> ("VISA resource name out"=w400:refnum<visa-resource-name>)  [unwired: 7 in, 1 out]
      n156 = call <instrlib>:"Configure Source (Level).vi"("VISA resource name"=w400, "Source Measure Unit Channel (0: Channel A)"=w402, "Level Type (1: Voltage)"=w402, "Voltage Level (0 V)"=w403) -> ("VISA resource name out"=w404:refnum<visa-resource-name>)  [unwired: 10 in, 1 out]
      n157 = call <instrlib>:"Enable Source Output.vi"("Output Mode (0: Turn off)"=w401, "Source Measure Unit Channel (0: Channel A)"=w402, "VISA resource name"=w404) -> ("VISA resource name out"=w399:refnum<visa-resource-name>)  [unwired: 7 in, 1 out]
      n158 = call <instrlib>:"Close.vi"("VISA resource name"=w399) -> ()  [unwired: 10 in, 1 out]
    }
  }
